vi "Display Module.vi"(7 "Callling VI":refnum<vi>) -> ()   [LabVIEW 2020]
uses:
  Display Module TypeDefs/IMAQ Z Scale Bar.ctl
  <vilib>/Utility/miscctls.llb/LVPointTypeDef.ctl
  <vilib>/vision/Image Controls.llb/IMAQ Image.ctl
  <vilib>/Utility/miscctls.llb/LVRectTypeDef.ctl
  Hardware Configuration/Hardware Configuration Controls/Standard Action.ctl
  <vilib>/event_ctls.llb/lveventtype.ctl
  Tools/TIFF Image Read and Write/ImageJ TIF Type Defs/TIF Write Image Information.ctl
  <vilib>/vision/NI_Vision_Development_Module.lvlib
panel:
  in  "Settings Menu":T1
  in  "Settings":bool
  in  "Refresh Rate (ms)":u32=30
  in  "Z Scale Channel 6":T2
  in  "Z Scale Channel 5":T2
  in  "Z Scale Channel 4":T2
  in  "Z Scale Channel 3":T2
  in  "Z Scale Channel 2":T2
  in  "Z Scale Channel 1":T2
  out "Messages":string
  in  "Max Left":bool
  in  "Max Right":bool
  in  "Add Display":bool
  in  "Remove Display":bool
  in  "Exit":bool
  out "Channel 6":T3(plugin-control)
  out "Channel 5":T3(plugin-control)
  out "Channel 4":T3(plugin-control)
  out "Channel 3":T3(plugin-control)
  out "Channel 2":T3(plugin-control)
  out "Channel 1":T3(plugin-control)
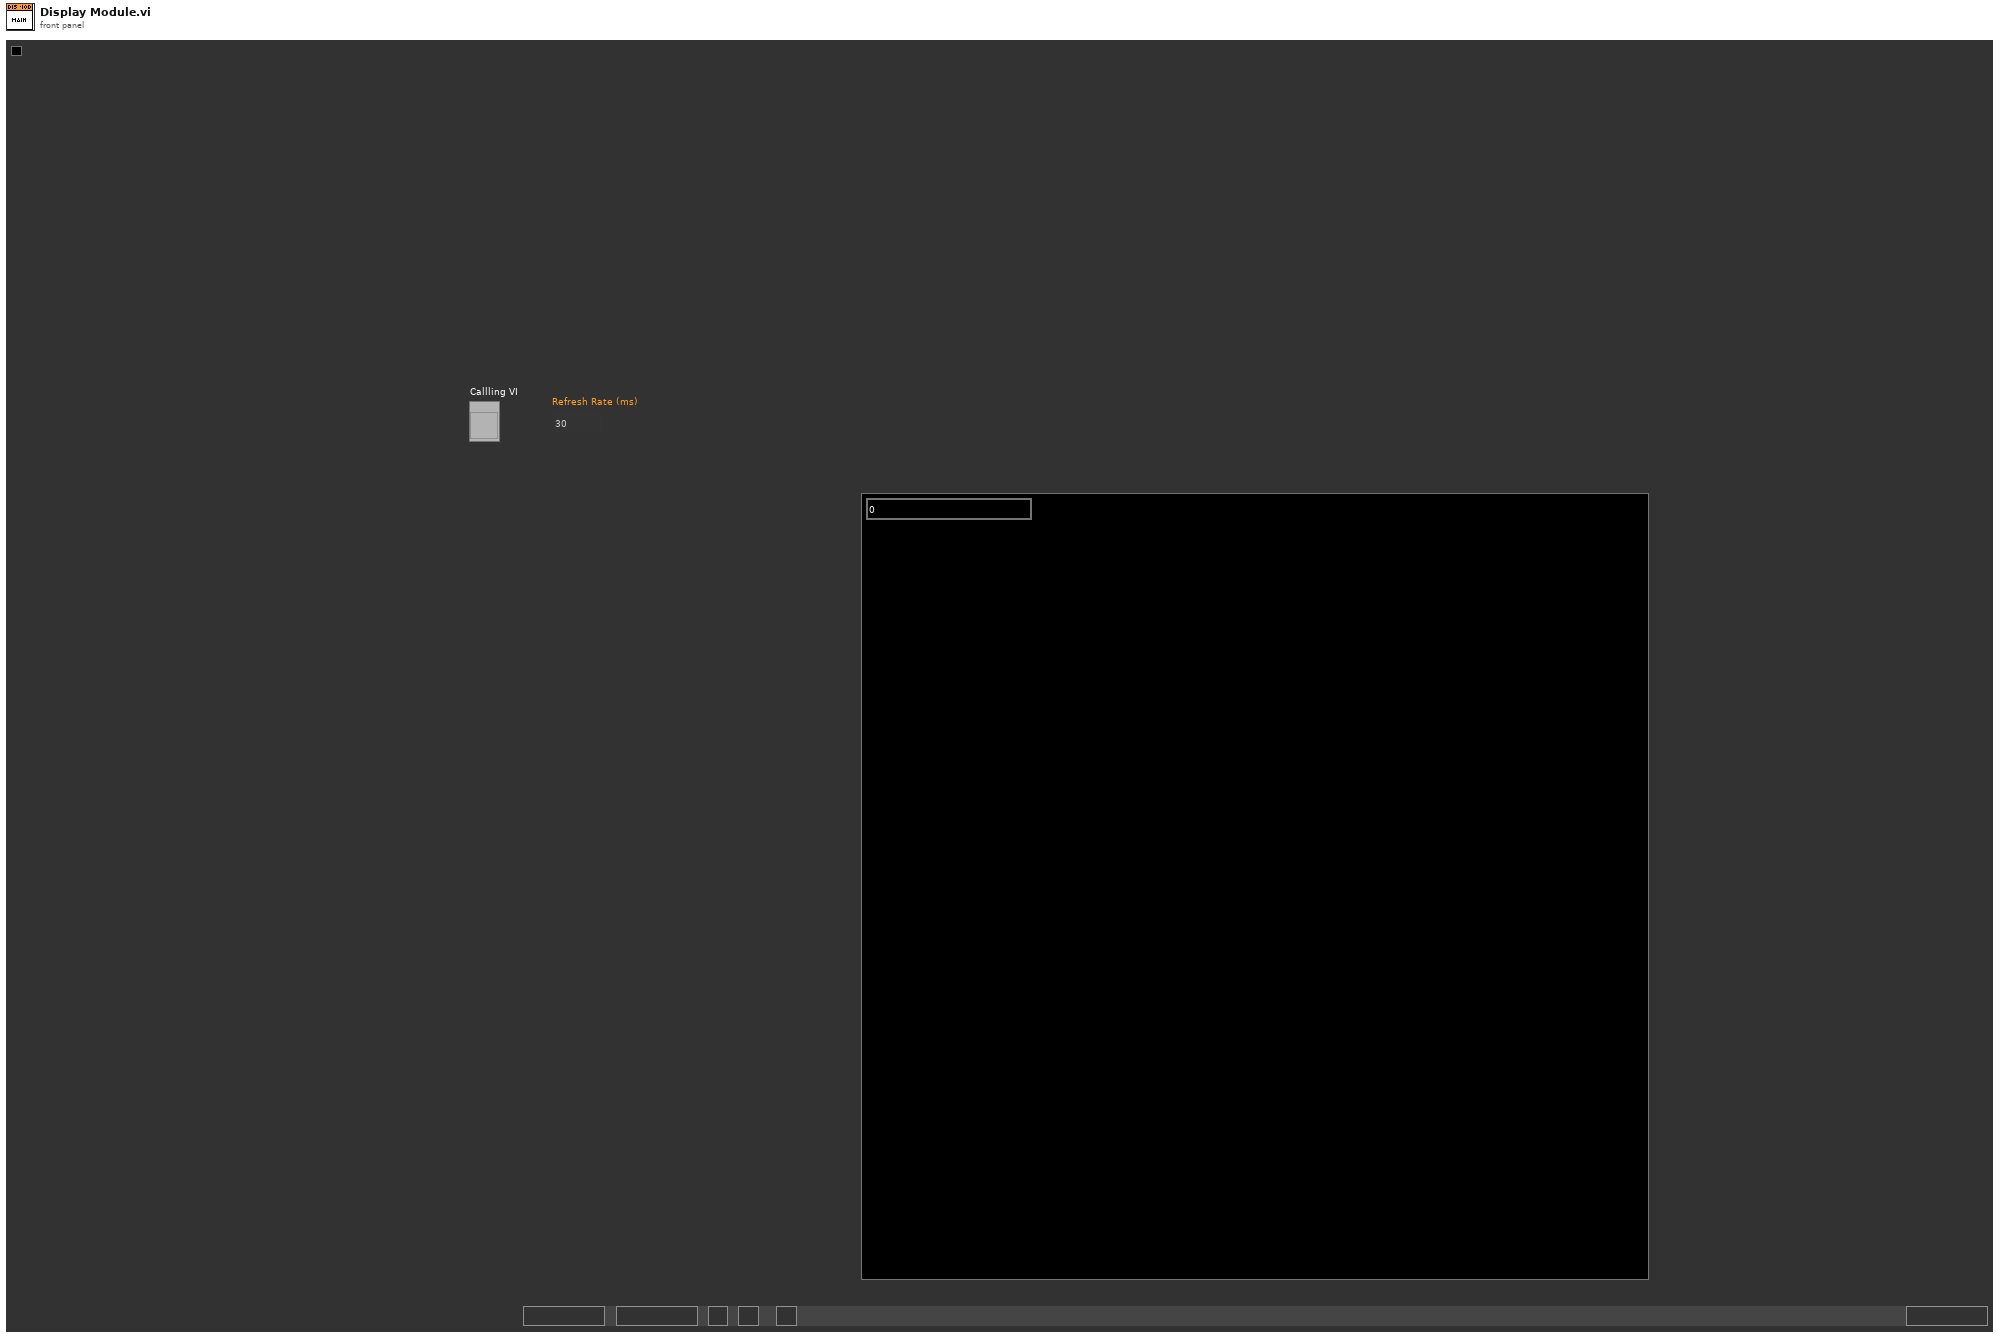
[diagram p1: front panel]
types:
  T1 = cluster{"Refresh Rate":bool, "Change Display Order":bool, "Display On / Off":bool}
  T2 = typedef "IMAQ Z Scale Bar.ctl" = cluster{"Z Scale Image":T3, "Z Scale Min":sgl, "Z Scale Max":sgl}
  T3 = typedef "IMAQ Image.ctl" = refnum<image>
  T4 = typedef "Image Type" = u32
  T5 = typedef "LVPointTypeDef.ctl" = cluster{"Horizontal":i16, "Vertical":i16}
  T6 = enum32{"Invalid", "Standard", "Closed", "Hidden", "Minimized", "Maximized"}
  T7 = enum16{"Always On", "Always Off", "Off While Running"}
  T8 = enum16{"Change Number", "Refresh Positions", "Get No. of Displays"}
  T9 = typedef "Standard Action.ctl" = enum16{"Read", "Write"}
  T10 = typedef "LVRectTypeDef.ctl" = cluster{"Left":i16, "Top":i16, "Right":i16, "Bottom":i16}
  T11 = typedef "lveventtype.ctl" = enum32{"Null", "Timeout", "Annotation Menu Selection", "Annotation Menu Selection?", "App Instance Close", "App Instance Close?", "Autoscale Range Change", "Bookmark Info Change", "Cell Edit", "Cell Edit?", "Cursor Grab", "Cursor Grab?", "Cursor Menu Selection", "Cursor Menu Selection?", "Cursor Move", "Cursor Release", "Data Change", "Direction Change", "Display State Change", "Drag Ended", "Drag Enter", "Drag Leave", "Drag Over", "Drag Source Update", "Drag Starting", "Drag Starting?", "Drop", "Exec State Change", "Key Down", "Key Down?", "Key Repeat", "Key Repeat?", "Key Up", "Listbox Double Click", "Menu Activation?", "Menu Selection (App)", "Menu Selection? (App)", "Menu Selection (User)", "Mouse Down", "Mouse Down?", "Mouse Enter", "Mouse Leave", "Mouse Move", "Mouse Up", "Mouse Wheel", "NI Security User Change (App)", "Pane Size", "Panel Close", "Panel Close?", "Panel Resize", "Plot Attribute Change", "Scale Range Change", "Shortcut Menu Activation?", "Shortcut Menu Selection (App)", "Shortcut Menu Selection? (App)", "Shortcut Menu Selection (User)", "Tree Double Click", "Tree Drag", "Tree Drag?", "Tree Drop", "Tree Drop?", "Tree Item Close", "Tree Item Close?", "Tree Item Open", "Tree Item Open?", "User Event", "Value Change"}
  T12 = cluster{"Global Rectangle":i32[], "Contours":cluster{"Contour Type":u32, "ROI Type":u32, "Points":i32[]}[]}
  T13 = typedef "TIF Write Image Information.ctl" = cluster{"Image Width (Pixels)":u32, "Image Height (Pixels)":u32, "Pixel Width (µm)":dbl, "Pixel Height (µm)":dbl, "Bits Per Sample (e.g. 16)":u32, "No. of Frames":u32, "No. of Slices":u32, "Time Step (sec)":dbl, "Z Step (µm)":dbl}
  T14 = typedef "LVAllMonitorsDisplayTypeDef.ctl" = cluster{"Bounds":cluster{"Left":i16, "Top":i16, "Right":i16, "Bottom":i16}, "Depth":i16}[]
  T15 = cluster{"Bounds":cluster{"Left":i16, "Top":i16, "Right":i16, "Bottom":i16}, "Depth":i16}
  T16 = cluster{"Mean Value":sgl, "Standard Variation":sgl, "Minimal Value":sgl, "Maximal Value":sgl, "Area (calibrated)":sgl, "Area (pixels)":u32, "%":sgl, "Calibration Valid":bool}
  T17 = enum16{"big-endian, network order", "native, host order", "little-endian"}
  T18 = cluster{"Contour Type":u32, "ROI Type":u32, "Points":i32[]}[]
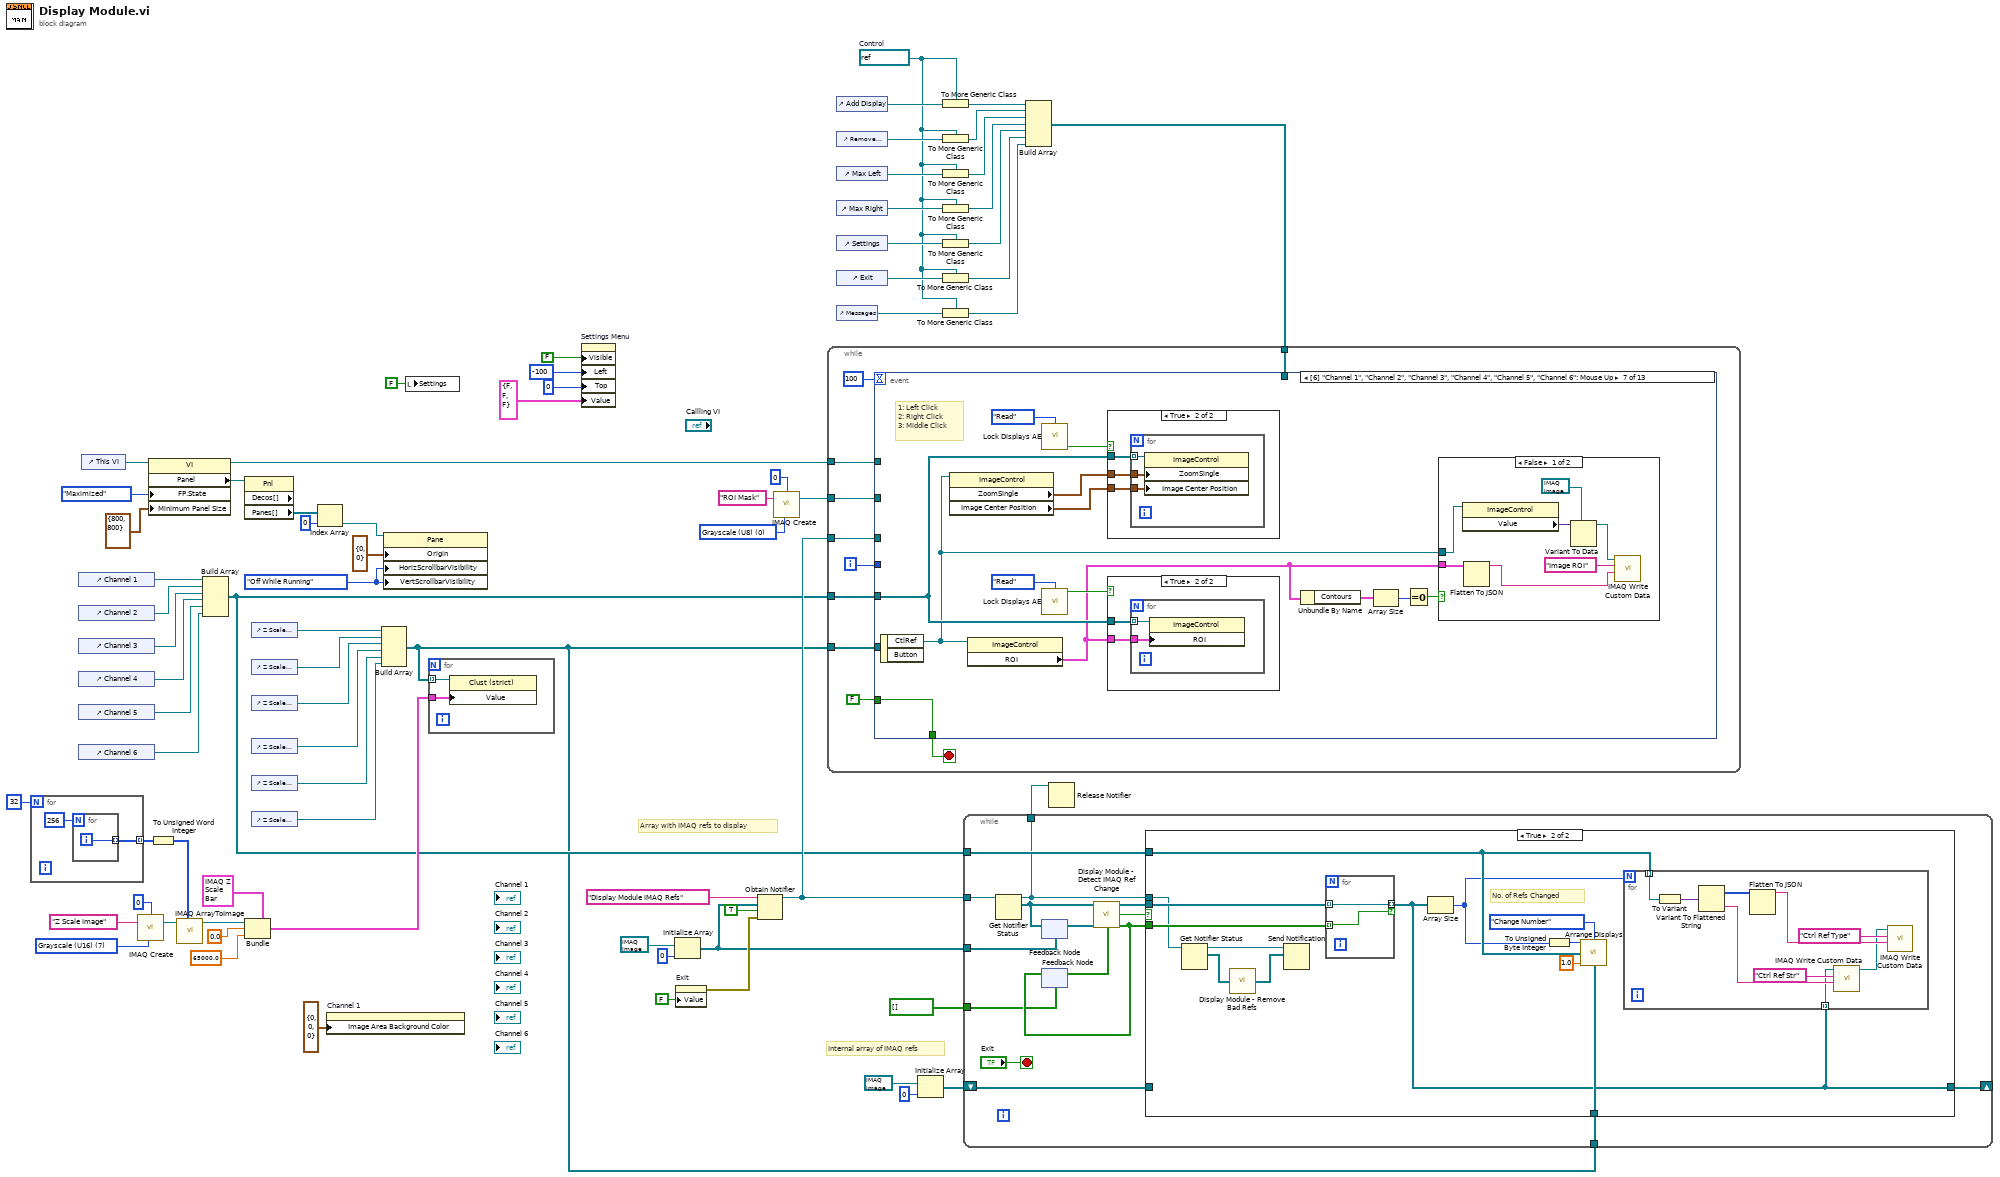
[diagram p0: block diagram]
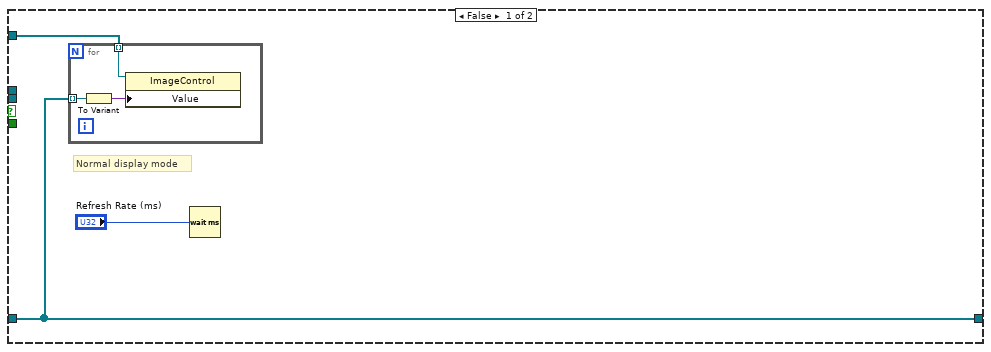
[diagram p2: hidden frame]
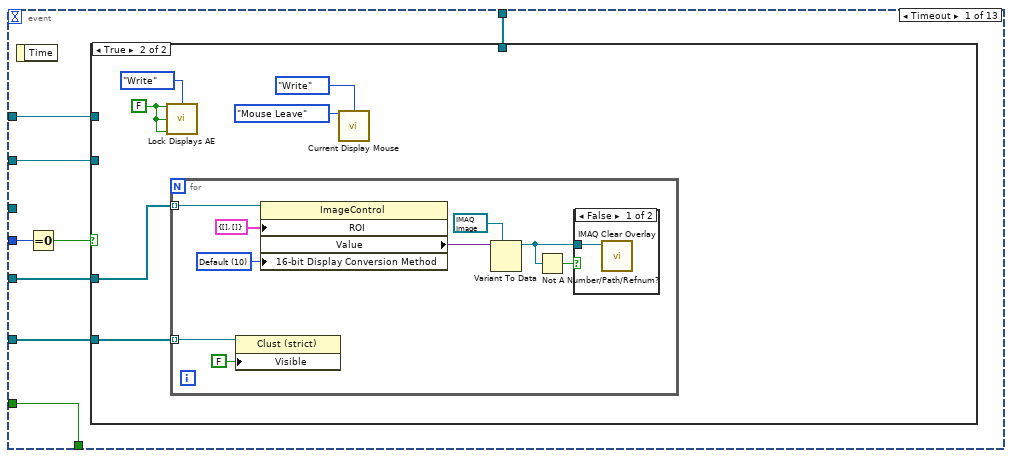
[diagram p3: hidden frame]
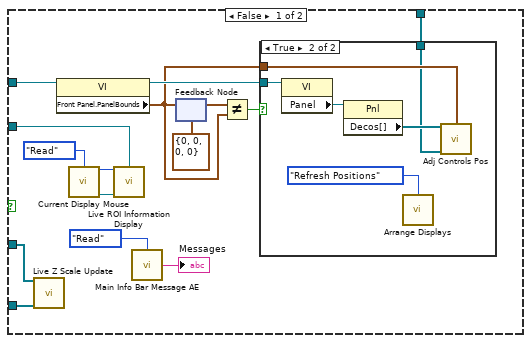
[diagram p4: hidden frame]
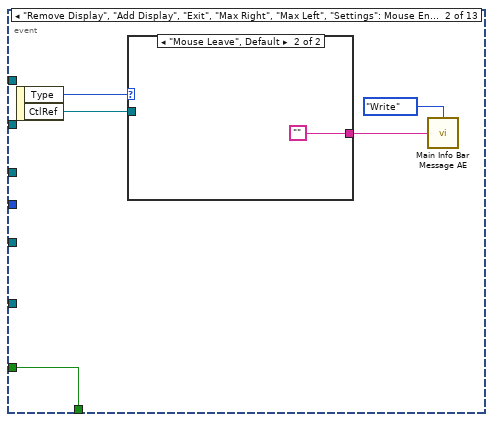
[diagram p7: hidden frame]
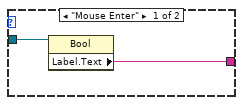
[diagram p8: hidden frame]
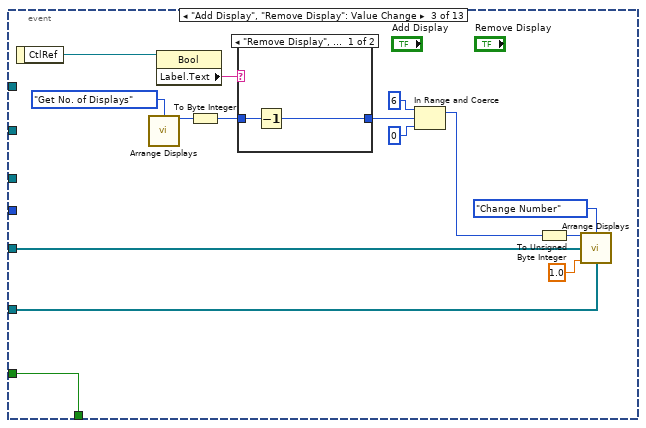
[diagram p9: hidden frame]
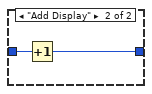
[diagram p10: hidden frame]
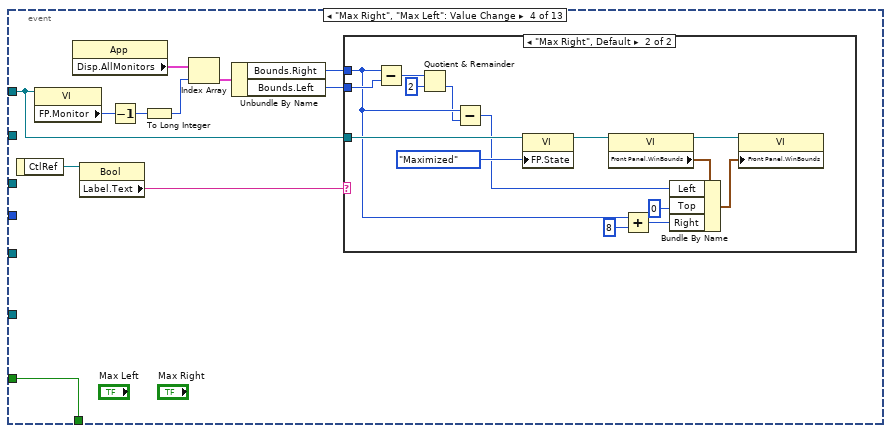
[diagram p11: hidden frame]
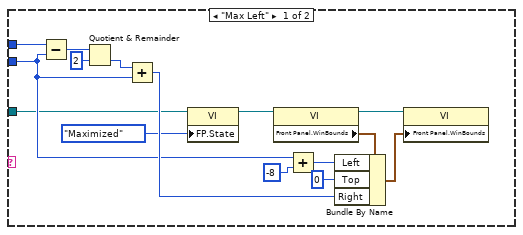
[diagram p12: hidden frame]
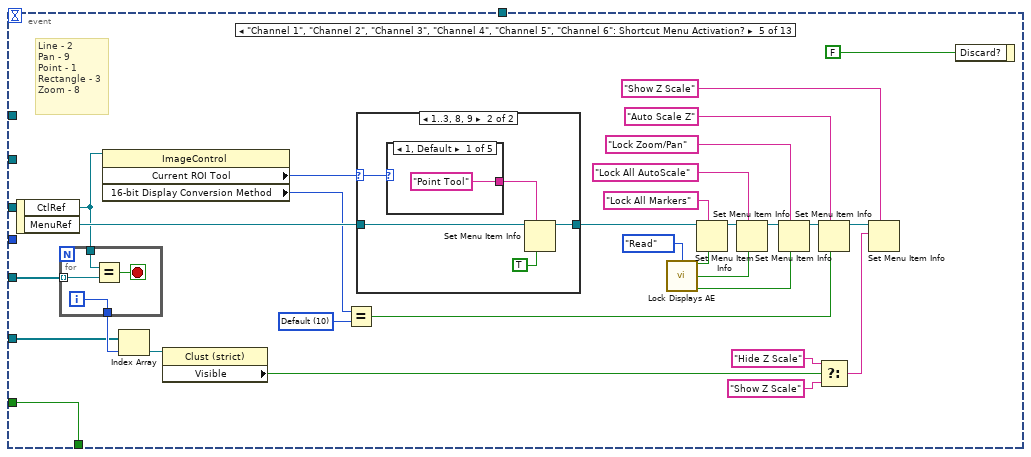
[diagram p13: hidden frame]
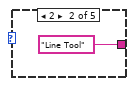
[diagram p15: hidden frame]
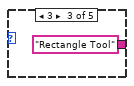
[diagram p16: hidden frame]
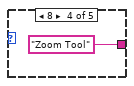
[diagram p17: hidden frame]
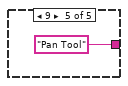
[diagram p18: hidden frame]
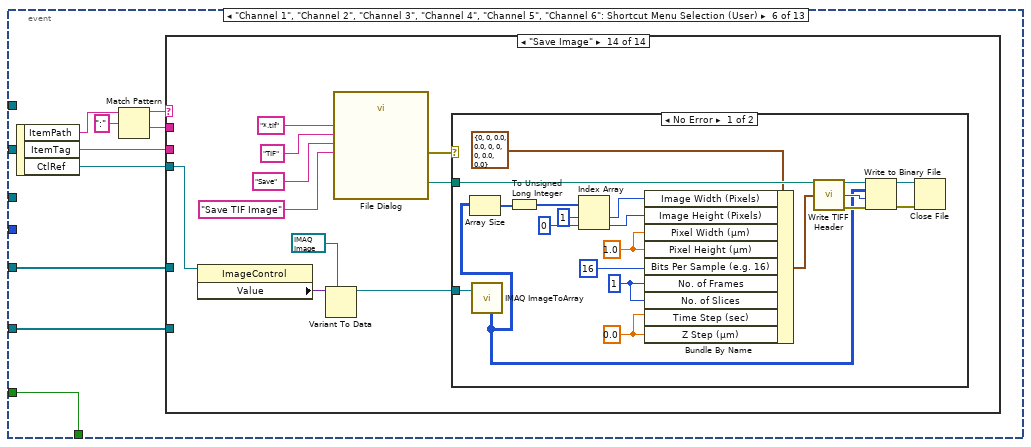
[diagram p19: hidden frame]
diagram:
  w23 = refnum<vi> refnum  # Control
  w47 = T4 7 items=["Grayscale (U8)", "Grayscale (I16)", "Grayscale (SGL)", "Complex (CSG)", "RGB (U32)", "HSL (U32)", "RGB (U64)", "Grayscale (U16)"] ("Image Type")
  w53 = T4 0 items=["Grayscale (U8)", "Grayscale (I16)", "Grayscale (SGL)", "Complex (CSG)", "RGB (U32)", "HSL (U32)", "RGB (U64)", "Grayscale (U16)"] ("Image Type")
  w66 = T7."Off While Running" ("Vertical Scrollbar Visibility")
  # "Internal array of IMAQ refs"
  # "Array with IMAQ refs to display"
  n1 = for {
    N: 32 -> [_]
    tunnel: [w76] -> w45 mode=indexing
    n2 = for {
      N: 256 -> [_]
      tunnel: [w78] -> w76 mode=indexing
      i -> [w78]
    }
  }
  n3 = control-ref of="Channel 1"() -> (w75:refnum<vi>)
  n4 = control-ref of="Channel 2"() -> (w70:refnum<vi>)
  n5 = control-ref of="Channel 3"() -> (w71:refnum<vi>)
  n6 = control-ref of="Channel 4"() -> (w72:refnum<vi>)
  n7 = control-ref of="Channel 5"() -> (w73:refnum<vi>)
  n8 = control-ref of="Channel 6"() -> (w74:refnum<vi>)
  n9 = control-ref of="This VI"() -> (w65:refnum<vi>)
  n10 = call "IMAQ Create"("Border Size"=0, "Image Name"="Z Scale Image", "Image Type"=w47) -> ("New Image"=w46:T3)  [unwired: 2 in, 1 out]
  n11 = property class="VI"(reference=w65, "FP.State"=T6."Maximized" ("Front Panel Window:State"), "Minimum Panel Size"=T5 {"Horizontal"=800, "Vertical"=800} ("Front Panel Window:Minimum Size")) -> (reference out=w60:refnum<vi>, "Panel"=w61:refnum<vi>)  [unwired: 1 in, 1 out]
  n12 = To Unsigned Word Integer(number=w45) -> (unsigned 16bit integer=w44:u16[][])
  n13 = call "IMAQ ArrayToImage"("Image Pixels (U16)"=w44, "Image"=w46) -> ("Image Out"=w43:T3)  [unwired: 8 in, 1 out]
  n14 = Build Array(w75, w70, w71, w72, w73, w74) -> (w3:refnum<vi>[])
  n15 = property class="Pnl" props=["Decos[]", "Panes[]"](reference=w61) -> ("Panes[]"=w62:refnum<vi>[])  [unwired: 1 in, 3 out]
  n16 = Bundle(cluster=T2 {"Z Scale Image"="remote image 000001BB3853FFD8", "Z Scale Min"=0.0, "Z Scale Max"=65000.0} ("Z Scale Channel 6"), "Z Scale Image"=w43, "Z Scale Min"=sgl 0.0, "Z Scale Max"=sgl 65000.0) -> (w35:T2)
  n17 = control-ref of="Z Scale Channel 1"() -> (w1:refnum<vi>)
  n18 = control-ref of="Z Scale Channel 2"() -> (w36:refnum<vi>)
  n19 = control-ref of="Z Scale Channel 3"() -> (w37:refnum<vi>)
  n20 = control-ref of="Z Scale Channel 4"() -> (w38:refnum<vi>)
  n21 = control-ref of="Z Scale Channel 5"() -> (w39:refnum<vi>)
  n22 = control-ref of="Z Scale Channel 6"() -> (w40:refnum<vi>)
  n23 = Index Array(array=w62, index=0) -> (element=w68:refnum<vi>)
  n24 = property on="Channel 1" class="ImageControl"("Image Area Background Color"=cluster{"Red":u8, "Green":u8, "Blue":u8} {"Red"=0, "Green"=0, "Blue"=0} ("Image Area:Background:Background Color")) -> ()  [unwired: 2 in, 2 out]
  n25 = Build Array(w1, w36, w37, w38, w39, w40) -> (w2:refnum<vi>[])
  n26 = property class="Pane"(reference=w68, "Origin"=T5 {"Horizontal"=0, "Vertical"=0}, "HorizScrollbarVisibility"=w66, "VertScrollbarVisibility"=w66) -> ()  [unwired: 1 in, 2 out]
  n27 = local write "Settings"(FALSE ("Settings")) -> ()
  n28 = for {
    tunnel: w2 -> [w80] mode=indexing
    tunnel: w35 -> [w79]
    n29 = property class="Clust (strict)"(reference=w80, "Value"=w79) -> ()  [unwired: 1 in, 2 out]
  }
  n30 = property on="Settings Menu" class="Clust (strict)"("Visible"=FALSE, "Left"=-100 ("Position:Left"), "Top"=0 ("Position:Top"), "Value"=T1 {"Refresh Rate"=FALSE, "Change Display Order"=FALSE, "Display On / Off"=FALSE} ("Settings Menu")) -> ()  [unwired: 2 in, 2 out]
  n31 = Initialize Array(T3 refnum ("New Image"), 0 ("dimension size")) -> (w6:T3[])
  n32 = property on="Exit" class="Bool (strict)"("Value"=FALSE ("Exit")) -> (error out=w31:errorcluster)  [unwired: 2 in, 1 out]
  n33 = Obtain Notifier(name (unnamed)="Display Module IMAQ Refs", notification data type=w6, create if not found? (T)=TRUE, error in (no error)=w31) -> (notifier out=w5:refnum<notifier>)  [unwired: 2 out]
  n34 = call "IMAQ Create"("Border Size"=0, "Image Name"="ROI Mask", "Image Type"=w53) -> ("New Image"=w51:T3)  [unwired: 2 in, 1 out]
  n35 = control-ref of="Add Display"() -> (w30:refnum<vi>)
  n36 = control-ref of="Remove Display"() -> (w24:refnum<vi>)
  n37 = control-ref of="Max Left"() -> (w25:refnum<vi>)
  n38 = control-ref of="Max Right"() -> (w26:refnum<vi>)
  n39 = control-ref of="Settings"() -> (w27:refnum<vi>)
  n40 = control-ref of="Exit"() -> (w28:refnum<vi>)
  n41 = control-ref of="Messages"() -> (w29:refnum<vi>)
  n42 = Initialize Array(T3 refnum ("New Image"), 0 ("dimension size")) -> (w7:T3[])
  n43 = To More Generic Class(target class=w23, reference=w30) -> (generic class reference=w22:refnum<vi>)
  n44 = To More Generic Class(target class=w23, reference=w24) -> (generic class reference=w21:refnum<vi>)
  n45 = To More Generic Class(target class=w23, reference=w25) -> (generic class reference=w20:refnum<vi>)
  n46 = To More Generic Class(target class=w23, reference=w26) -> (generic class reference=w19:refnum<vi>)
  n47 = To More Generic Class(target class=w23, reference=w27) -> (generic class reference=w18:refnum<vi>)
  n48 = To More Generic Class(target class=w23, reference=w28) -> (generic class reference=w17:refnum<vi>)
  n49 = To More Generic Class(target class=w23, reference=w29) -> (generic class reference=w16:refnum<vi>)
  n50 = while {
    tunnel: w5 -> [w95]
    tunnel: w3 -> [w94]
    tunnel: [w84] -> w55
    tunnel: w2 -> [w92]
    shift-right: [w85] -> _
    shift-left: w7 -> [w91]
    tunnel: w6 -> [w88]
    tunnel: bool[] [] -> [w81]
    stop <- "Exit" stop-if-true
    n51 = Get Notifier Status(notifier=w95) -> (notifier out=w84:refnum<notifier>, current notification=w90:T3[])  [unwired: 1 in, 3 out]
    n52 = feedback-in #1(w90) -> ()
    n53 = feedback #1(w88) -> (w89:T3[])
    n54 = feedback #2(w81) -> (w82:bool[])
    n55 = call "Display Module - Detect IMAQ Ref Change.vi"("Current Image Refs"=w90, "Previous Image Refs"=w89, "Previous Image Display Flags"=w82) -> ("Current Image Refs (Dup)"=w87:T3[], "Change Detected"=w86:bool, "Image Display Flags"=w83:bool[])  [unwired: 10 in]
    n56 = feedback-in #2(w83) -> ()
    n57 = case shown="True" w86 {
      tunnel: w87 -> [_ w110]
      tunnel: w94 -> [w98 w104]
      tunnel: w92 -> [_ w112]
      tunnel: w91 -> [w96 _]
      tunnel: w83 -> [_ w109]
      tunnel: [w96 w102] -> w85
      tunnel: w84 -> [_ w105]
      frame False {
        # "Normal display mode"
        n58 = for {
          tunnel: w98 -> [w101] mode=indexing
          tunnel: w96 -> [w99] mode=indexing
          n59 = To Variant(anything=w99) -> (Variant=w100:variant)
          n60 = property class="ImageControl"(reference=w101, "Value"=w100) -> ()  [unwired: 1 in, 2 out]
        }
        n61 = Wait (ms)(milliseconds to wait="Refresh Rate (ms)") -> ()  [unwired: 1 out]
      }
      frame True {
        # "No. of Refs Changed"
        n62 = Get Notifier Status(notifier=w105) -> (notifier out=w107:refnum<notifier>, current notification=w106:T3[])  [unwired: 1 in, 3 out]
        n63 = call "Display Module - Remove Bad Refs.vi"("Image Refs In"=w106) -> ("Image Refs Out"=w108:T3[])  [unwired: 14 in]
        n64 = Send Notification(notification=w108, notifier=w107) -> ()  [unwired: 1 in, 2 out]
        n65 = for {
          tunnel: w110 -> [w125] mode=indexing
          tunnel: [w125] -> w102 mode=indexing if=w124
          tunnel: w109 -> [w124] mode=indexing
        }
        n66 = Array Size(array=w102) -> (size(s)=w103:i32)
        n67 = To Unsigned Byte Integer(number=w103) -> (unsigned 8bit integer=w114:u8)
        n68 = call "Arrange Displays.vi"("Number of Displays"=w114, "Action"=T8."Change Number", "IMAQ Display Refs"=w104, "Aspect Ratio (Width/Height)"=1.0, "Z Scale Refs"=w112) -> ()  [unwired: 9 in, 2 out]
        n69 = for {
          N: w103 -> [_]
          tunnel: w104 -> [w122] mode=indexing
          tunnel: w102 -> [w115] mode=indexing
          n70 = To Variant(anything=w122) -> (Variant=w123:variant)
          n71 = Variant To Flattened String(Variant=w123) -> (data string=w117:string, 1:w120:i16[])
          n72 = Flatten To JSON(anything=w120) -> (JSON string=w118:string)  [unwired: 2 in, 1 out]
          n73 = call "IMAQ Write Custom Data"("Custom Data In"=w117, "Key"="Ctrl Ref Str", "Image"=w115) -> ("Image Out"=w116:T3)  [unwired: 7 in, 1 out]
          n74 = call "IMAQ Write Custom Data"("Custom Data In"=w118, "Key"="Ctrl Ref Type", "Image"=w116) -> ()  [unwired: 7 in, 2 out]
        }
      }
    }
  }
  n75 = Build Array(w22, w21, w20, w19, w18, w17, w16) -> (w15:refnum<vi>[])
  n76 = while {
    tunnel: w3 -> [w134]
    tunnel: w60 -> [w130]
    tunnel: w51 -> [w129]
    tunnel: w2 -> [w128]
    tunnel: w15 -> [w127]
    tunnel: w5 -> [w126]
    i -> [w135]
    stop <- w133 stop-if-true
    n77 = event shown="[6] \"Channel 1\", \"Channel 2\", \"Channel 3\", \"Channel 4\", \"Channel 5\", \"Channel 6\": Mouse Up" {
      selector: _ -> [_ _ _ _ _ _ _ _ _ _ _ _ _]
      dyn-events: _ -> [_ _ _ _ _ _ _ _ _ _ _ _ _]
      timeout: 100 -> [_ _ _ _ _ _ _ _ _ _ _ _ _]
      tunnel: w135 -> [w143 _ _ _ _ _ _ _ _ _ _ _ _]
      tunnel: w134 -> [w141 _ w190 _ w253 w296 w496 _ w532 w540 _ w567 w603]
      tunnel: [w140 w185 w203 w218 w277 w302 w501 w523 w534 w546 w556 w579 w604] -> w133
      tunnel: FALSE -> [w140 w185 w203 w218 w277 w302 w501 w523 w534 w546 w556 w579 _]
      tunnel: w130 -> [w139 _ _ w209 _ _ _ _ _ _ _ _ _]
      tunnel: w129 -> [w138 _ _ _ _ _ _ _ _ _ _ _ w602]
      tunnel: w128 -> [w137 _ w191 _ w254 w295 _ _ w533 _ _ _ _]
      tunnel: w127 -> [w136 _ _ _ _ _ _ _ _ _ _ _ _]
      tunnel: w126 -> [_ _ _ _ _ _ _ _ _ _ _ w568 _]
      event Timeout {
        n78 = event-data() -> ()  [unwired: 1 in, 1 out]
        n79 = Equal To 0?(x=w143) -> (x = 0?=w142:bool)
        n80 = case shown="True" w142 {
          tunnel: w141 -> [w146 w168]
          tunnel: w139 -> [w158 _]
          tunnel: w138 -> [w152 _]
          tunnel: w137 -> [w145 w167]
          tunnel: w136 -> [w144 _]
          frame False {
            n81 = call "Live Z Scale Update.vi"("IMAQ Display Refs"=w146, "Z Scale Refs"=w145) -> ()  [unwired: 14 in]
            n82 = property class="VI"(reference=w158) -> (reference out=w154:refnum<vi>, "Front Panel.PanelBounds"=w153:T10)  [unwired: 1 in, 1 out]
            n83 = call "Current Display Mouse.vi"("Action"=Standard_Action."Read") -> ("Event Type Out"=w150:T11, "IMAQ Image Display Ref Out"=w149:refnum<vi>)  [unwired: 13 in]
            n84 = call "Live ROI Information Display.vi"("Event Type"=w150, "ROI Mask REF"=w152, "IMAQ Image Display Ref"=w149) -> ()  [unwired: 13 in]
            n85 = call "Main Info Bar Message AE.vi"("Action"=Standard_Action."Read") -> ("Message Out"=→"Messages":string)  [unwired: 14 in]
            n86 = feedback-in #3(w153) -> ()
            n87 = feedback #3(T10 {"Left"=0, "Top"=0, "Right"=0, "Bottom"=0} ("Front Panel.PanelBounds")) -> (w157:T10)
            n88 = Not Equal?(x=w157, y=w153) -> (x != y?=w155:bool)
            n89 = case shown="True" w155 {
              tunnel: w154 -> [_ w162]
              tunnel: w153 -> [_ w161]
              tunnel: w144 -> [_ w160]
              frame False {
              }
              frame True {
                n90 = property class="VI"(reference=w162) -> ("Panel"=w164:refnum<vi>)  [unwired: 1 in, 2 out]
                n91 = property class="Pnl"(reference=w164) -> ("Decos[]"=w163:refnum<vi>[])  [unwired: 1 in, 2 out]
                n92 = call "Arrange Displays.vi"("Action"=T8."Refresh Positions") -> ()  [unwired: 13 in, 2 out]
                n93 = call "Adj Controls Pos.vi"("Decoration Ref Array"=w163, "Panel Bounds"=w161, "Control Ref Array"=w160) -> ()  [unwired: 13 in]
              }
            }
          }
          frame True {
            w170 = FALSE ("Lock All Markers")
            n94 = call "Lock Displays AE.vi"("Lock All Markers"=w170, "Action"=Standard_Action."Write", "Lock All AutoScale"=w170, "Lock Pan/Zoom"=w170) -> ()  [unwired: 9 in, 3 out]
            n95 = for {
              tunnel: w168 -> [w174] mode=indexing
              tunnel: w167 -> [w173] mode=indexing
              w171 = u32 10 items=["Default"=10, "Most Significant Bits"=11, "Full Dynamic"=12, "Downshift"=13, "Given Range"=14, "90% Dynamic"=15, "Given Percent Range"=16] ("16-bit Display Mapping:Conversion Method")
              n96 = property class="Clust (strict)"(reference=w173, "Visible"=FALSE) -> ()  [unwired: 1 in, 2 out]
              n97 = property class="ImageControl"(reference=w174, "ROI"=T12 {"Global Rectangle"=[], "Contours"=[]}, "16-bit Display Conversion Method"=w171) -> ("Value"=w175:variant)  [unwired: 1 in, 2 out]
              n98 = Variant To Data(type=T3 refnum ("New Image"), Variant=w175) -> (data=w178:T3)  [unwired: 1 in, 1 out]
              n99 = Not A Number/Path/Refnum?(number/path/refnum=w178) -> (NaN/Path/Refnum?=w177:bool)
              n100 = case shown="False" w177 {
                tunnel: w178 -> [w180 _]
                frame False {
                  n101 = call "IMAQ Clear Overlay"("Image"=w180) -> ()  [unwired: 9 in, 2 out]
                }
                frame True {
                }
              }
            }
            n102 = call "Current Display Mouse.vi"("Event Type"=lveventtype."Mouse Leave", "Action"=Standard_Action."Write") -> ()  [unwired: 12 in, 2 out]
          }
        }
      }
      event "Remove Display", "Add Display", "Exit", "Max Right", "Max Left", "Settings", "Settings Menu.Refresh Rate", "Settings Menu.Change Display Order", "Settings Menu.Display On / Off": Mouse Enter; "Remove Display", "Add Display", "Exit", "Max Right", "Max Left", "Settings", "Settings Menu.Refresh Rate", "Settings Menu.Change Display Order", "Settings Menu.Display On / Off": Mouse Leave {
        n103 = event-data() -> ("Type"=w184:T11, "CtlRef"=w183:refnum<vi>)  [unwired: 1 in]
        n104 = case shown="\"Mouse Leave\", Default" w184 {
          tunnel: w183 -> [w187 _]
          tunnel: [w186 ""] -> w181
          frame "Mouse Enter" {
            n105 = property class="Bool"(reference=w187) -> ("Label.Text"=w186:string)  [unwired: 1 in, 2 out]
          }
          frame "Mouse Leave", Default {
          }
        }
        n106 = call "Main Info Bar Message AE.vi"("Action"=Standard_Action."Write", "Message"=w181) -> ()  [unwired: 13 in, 1 out]
      }
      event "Add Display", "Remove Display": Value Change {
        n107 = event-data() -> ("CtlRef"=w202:refnum<vi>)  [unwired: 1 in]
        n108 = call "Arrange Displays.vi"("Action"=T8."Get No. of Displays") -> ("Number of Displays Out"=w193:u8)  [unwired: 13 in, 1 out]
        n109 = property class="Bool"(reference=w202) -> ("Label.Text"=w201:string)  [unwired: 1 in, 2 out]
        n110 = To Byte Integer(number=w193) -> (8bit integer=w192:i8)
        n111 = case shown="\"Remove Display\", Default" w201 {
          tunnel: w192 -> [w205 w207]
          tunnel: [w204 w206] -> w198
          frame "Remove Display", Default {
            n112 = Decrement(x=w205) -> (x-1=w204:i8)
          }
          frame "Add Display" {
            n113 = Increment(x=w207) -> (x+1=w206:i8)
          }
        }
        n114 = In Range and Coerce(upper limit=i8 6, x=w198, lower limit=i8 0) -> (coerced(x)=w197:i8)  [unwired: 1 out]
        n115 = To Unsigned Byte Integer(number=w197) -> (unsigned 8bit integer=w196:u8)
        n116 = call "Arrange Displays.vi"("Number of Displays"=w196, "Action"=T8."Change Number", "IMAQ Display Refs"=w190, "Aspect Ratio (Width/Height)"=1.0, "Z Scale Refs"=w191) -> ()  [unwired: 9 in, 2 out]
      }
      event "Max Right", "Max Left": Value Change {
        n117 = event-data() -> ("CtlRef"=w217:refnum<vi>)  [unwired: 1 in]
        n118 = property class="VI"(reference=w209) -> ("FP.Monitor"=w216:u16)  [unwired: 1 in, 2 out]
        n119 = property class="App"() -> ("Disp.AllMonitors"=w215:T14)  [unwired: 2 in, 2 out]
        n120 = property class="Bool"(reference=w217) -> ("Label.Text"=w208:string)  [unwired: 1 in, 2 out]
        n121 = Decrement(x=w216) -> (x-1=w214:u16)
        n122 = To Long Integer(number=w214) -> (32bit integer=w213:i32)
        n123 = Index Array(array=w215, index=w213) -> (element=w212:T15)
        n124 = Unbundle By Name(w212) -> ("Bounds.Right"=w211:i16, "Bounds.Left"=w210:i16)
        n125 = case shown="\"Max Right\", Default" w208 {
          tunnel: w211 -> [w233 w236]
          tunnel: w210 -> [w221 w240]
          tunnel: w209 -> [w219 w239]
          frame "Max Left" {
            n126 = Subtract(x=w233, y=w221) -> (x-y=w228:i16)
            n127 = Quotient & Remainder(x=w228, y=i16 2) -> (floor(x/y)=w226:i16)  [unwired: 1 out]
            n128 = Add(x=w226, y=w221) -> (x+y=w225:i16)
            n129 = property class="VI"(reference=w219, "FP.State"=T6."Maximized" ("Front Panel Window:State")) -> (reference out=w223:refnum<vi>)  [unwired: 1 in, 1 out]
            n130 = property class="VI"(reference=w223) -> (reference out=w232:refnum<vi>, "Front Panel.WinBounds"=w230:T10)  [unwired: 1 in, 1 out]
            n131 = Add(x=w221, y=i16 -8 ("Left")) -> (x+y=w220:i16)
            n132 = Bundle By Name(cluster=w230, "Left"=w220, "Top"=i16 0, "Right"=w225) -> (w231:T10)
            n133 = property class="VI"(reference=w232, "Front Panel.WinBounds"=w231) -> ()  [unwired: 1 in, 2 out]
          }
          frame "Max Right", Default {
            n134 = Subtract(x=w236, y=w240) -> (x-y=w245:i16)
            n135 = Quotient & Remainder(x=w245, y=i16 2) -> (floor(x/y)=w235:i16)  [unwired: 1 out]
            n136 = Subtract(x=w236, y=w235) -> (x-y=w234:i16)
            n137 = property class="VI"(reference=w239, "FP.State"=T6."Maximized" ("Front Panel Window:State")) -> (reference out=w242:refnum<vi>)  [unwired: 1 in, 1 out]
            n138 = property class="VI"(reference=w242) -> (reference out=w248:refnum<vi>, "Front Panel.WinBounds"=w246:T10)  [unwired: 1 in, 1 out]
            n139 = Add(x=w236, y=i16 8 ("Left")) -> (x+y=w237:i16)
            n140 = Bundle By Name(cluster=w246, "Left"=w234, "Top"=i16 0, "Right"=w237) -> (w247:T10)
            n141 = property class="VI"(reference=w248, "Front Panel.WinBounds"=w247) -> ()  [unwired: 1 in, 2 out]
          }
        }
      }
      event "Channel 1", "Channel 2", "Channel 3", "Channel 4", "Channel 5", "Channel 6": Shortcut Menu Activation? {
        w260 = u32 10 items=["Default"=10, "Most Significant Bits"=11, "Full Dynamic"=12, "Downshift"=13, "Given Range"=14, "90% Dynamic"=15, "Given Percent Range"=16] ("16-bit Display Mapping:Conversion Method")
        # "Line - 2\nPan - 9\nPoint - 1\nRectangle - 3\nZoom - 8"
        n142 = event-data() -> ("CtlRef"=w255:refnum<vi>, "MenuRef"=w275:refnum<k9>)  [unwired: 1 in]
        n143 = for {
          tunnel: w253 -> [w282] mode=indexing
          tunnel: w255 -> [w280]
          tunnel: [w279] -> w257
          i -> [w279]
          stop <- w281 stop-if-true
          n144 = Equal?(x=w280, y=w282) -> (x = y?=w281:bool)
        }
        n145 = property class="ImageControl"(reference=w255) -> ("Current ROI Tool"=w276:u32, "16-bit Display Conversion Method"=w262:u32)  [unwired: 1 in, 2 out]
        n146 = Index Array(array=w254, index=w257) -> (element=w256:refnum<vi>)
        n147 = property class="Clust (strict)"(reference=w256) -> ("Visible"=w249:bool)  [unwired: 1 in, 2 out]
        n148 = Equal?(x=w262, y=w260) -> (x = y?=w261:bool)
        n149 = case shown="1..3, 8, 9" w276 {
          selector: w276 -> [_ w288]
          tunnel: w275 -> [w283 w286]
          tunnel: [w283 w284] -> w274
          frame Default {
          }
          frame 1..3, 8, 9 {
            n150 = case shown="1, Default" w288 {
              tunnel: ["Point Tool" ("item tag") "Line Tool" ("item tag") "Rectangle Tool" ("item tag") "Zoom Tool" ("item tag") "Pan Tool" ("item tag")] -> w285
              frame 1, Default {
              }
              frame 2 {
              }
              frame 3 {
              }
              frame 8 {
              }
              frame 9 {
              }
            }
            n151 = Set Menu Item Info(6:TRUE ("checked"), 7:w285, 11:w286) -> (3:w284:refnum<k9>)  [unwired: 4 in, 1 out]
          }
        }
        n152 = call "Lock Displays AE.vi"("Action"=Standard_Action."Read") -> ("Lock All Markers Out"=w267:bool, "Lock All AutoScale Out"=w266:bool, "Lock Pan/Zoom Out"=w265:bool)  [unwired: 12 in]
        n153 = Set Menu Item Info(6:w267, 7:"Lock All Markers" ("item tag"), 11:w274) -> (3:w273:refnum<k9>)  [unwired: 4 in, 1 out]
        n154 = Set Menu Item Info(6:w266, 7:"Lock All AutoScale" ("item tag"), 11:w273) -> (3:w272:refnum<k9>)  [unwired: 4 in, 1 out]
        n155 = Set Menu Item Info(6:w265, 7:"Lock Zoom/Pan" ("item tag"), 11:w272) -> (3:w264:refnum<k9>)  [unwired: 4 in, 1 out]
        n156 = Set Menu Item Info(6:w261, 7:"Auto Scale Z" ("item tag"), 11:w264) -> (3:w259:refnum<k9>)  [unwired: 4 in, 1 out]
        n157 = Select(t="Hide Z Scale" ("item tag"), s=w249, f="Show Z Scale" ("item tag")) -> (s? t:f=w250:string)
        n158 = Set Menu Item Info(7:"Show Z Scale" ("item tag"), 10:w250, 11:w259) -> ()  [unwired: 4 in, 2 out]
        n159 = event-data("Discard?"=FALSE) -> ()  [unwired: 1 in, 1 out]
      }
      event "Channel 1", "Channel 2", "Channel 3", "Channel 4", "Channel 5", "Channel 6": Shortcut Menu Selection (User) {
        n160 = event-data() -> ("ItemPath"=w300:string, "ItemTag"=w301:string, "CtlRef"=w297:refnum<vi>)  [unwired: 1 in]
        n161 = Match Pattern(string=w300, regular expression=":") -> (before substring=w298:string, after substring=w294:string)  [unwired: 1 in, 2 out]
        n162 = case shown="\"Save Image\"" w298 {
          selector: w298 -> [_ _ w335 _ _ _ _ _ _ w431 _ _ _ _]
          tunnel: w297 -> [_ w315 w341 w366 _ w388 _ w402 w412 w429 w453 _ _ w462]
          tunnel: w301 -> [_ _ _ _ _ _ _ _ _ _ _ _ _ _]
          tunnel: w296 -> [_ w316 _ w369 w380 w390 _ w401 w413 w427 w449 _ _ _]
          tunnel: w295 -> [_ w314 _ w368 _ w389 _ _ _ _ _ _ _ _]
          tunnel: w294 -> [_ w303 _ _ _ _ _ _ _ _ _ _ _ _]
          frame Default {
          }
          frame "Color Map" {
            w309 = refnum<vi> refnum  # ImageControl
            w305 = u32 5 items=["Grayscale", "Binary", "Gradient", "Rainbow", "Temperature", "User Defined", "Binary 16 Bit", "Gradient 16 Bit", "Rainbow 16 Bit", "Temperature 16 Bit", "User Defined 16 Bit"] ("Palette:Palette Type")
            n163 = for {
              tunnel: w316 -> [w332] mode=indexing
              tunnel: [w333] -> w313
              tunnel: w315 -> [w331]
              i -> [w333]
              stop <- w330 stop-if-true
              n164 = Equal?(x=w331, y=w332) -> (x = y?=w330:bool)
            }
            n165 = Index Array(array=w314, index=w313) -> (element=w312:refnum<vi>)
            n166 = property class="Clust (strict)"(reference=w312) -> ("Controls[]"=w311:refnum<vi>[])  [unwired: 1 in, 2 out]
            n167 = property class="ImageControl"(reference=w315, "Palette Type"=w305) -> (reference out=w317:refnum<vi>)  [unwired: 1 in, 1 out]
            n168 = Index Array(array=w311, index=0) -> (element=w308:refnum<vi>)
            n169 = case shown="\"Glow\"" w303 {
              tunnel: [cluster{u8, u8, u8}[] [{0, 0, 0}, {1, 1, 1}, {2, 2, 2}, {3, 3, 3}, {4, 4, 4}, {5, 5, 5}, {6, 6, 6}, {7, 7, 7}, {8, 8, 8}, {9, 9, 9}, {10, 10, 10}, {11, 11, 11}, {12, 12, 12}, {13, 13, 13}, {14, 14, 14}, {15, 15, 15}, {16, 16, 16}, {17, 17, 17}, {18, 18, 18}, {19, 19, 19}, {20, 20, 20}, {21, 21, 21}, {22, 22, 22}, {23, 23, 23}, {24, 24, 24}, {25, 25, 25}, {26, 26, 26}, {27, 27, 27}, {28, 28, 28}, {29, 29, 29}, {30, 30, 30}, {31, 31, 31}, {32, 32, 32}, {33, 33, 33}, {34, 34, 34}, {35, 35, 35}, {36, 36, 36}, {37, 37, 37}, {38, 38, 38}, {39, 39, 39}, {40, 40, 40}, {41, 41, 41}, {42, 42, 42}, {43, 43, 43}, {44, 44, 44}, {45, 45, 45}, {46, 46, 46}, {47, 47, 47}, {48, 48, 48}, {49, 49, 49}, {50, 50, 50}, {51, 51, 51}, {52, 52, 52}, {53, 53, 53}, {54, 54, 54}, {55, 55, 55}, {56, 56, 56}, {57, 57, 57}, {58, 58, 58}, {59, 59, 59}, {60, 60, 60}, {61, 61, 61}, {62, 62, 62}, {63, 63, 63}, {64, 64, 64}, {65, 65, 65}, {66, 66, 66}, {67, 67, 67}, {68, 68, 68}, {69, 69, 69}, {70, 70, 70}, {71, 71, 71}, {72, 72, 72}, {73, 73, 73}, {74, 74, 74}, {75, 75, 75}, {76, 76, 76}, {77, 77, 77}, {78, 78, 78}, {79, 79, 79}, {80, 80, 80}, {81, 81, 81}, {82, 82, 82}, {83, 83, 83}, {84, 84, 84}, {85, 85, 85}, {86, 86, 86}, {87, 87, 87}, {88, 88, 88}, {89, 89, 89}, {90, 90, 90}, {91, 91, 91}, {92, 92, 92}, {93, 93, 93}, {94, 94, 94}, {95, 95, 95}, {96, 96, 96}, {97, 97, 97}, {98, 98, 98}, {99, 99, 99}, {100, 100, 100}, {101, 101, 101}, {102, 102, 102}, {103, 103, 103}, {104, 104, 104}, {105, 105, 105}, {106, 106, 106}, {107, 107, 107}, {108, 108, 108}, {109, 109, 109}, {110, 110, 110}, {111, 111, 111}, {112, 112, 112}, {113, 113, 113}, {114, 114, 114}, {115, 115, 115}, {116, 116, 116}, {117, 117, 117}, {118, 118, 118}, {119, 119, 119}, {120, 120, 120}, {121, 121, 121}, {122, 122, 122}, {123, 123, 123}, {124, 124, 124}, {125, 125, 125}, {126, 126, 126}, {127, 127, 127}, {128, 128, 128}, {129, 129, 129}, {130, 130, 130}, {131, 131, 131}, {132, 132, 132}, {133, 133, 133}, {134, 134, 134}, {135, 135, 135}, {136, 136, 136}, {137, 137, 137}, {138, 138, 138}, {139, 139, 139}, {140, 140, 140}, {141, 141, 141}, {142, 142, 142}, {143, 143, 143}, {144, 144, 144}, {145, 145, 145}, {146, 146, 146}, {147, 147, 147}, {148, 148, 148}, {149, 149, 149}, {150, 150, 150}, {151, 151, 151}, {152, 152, 152}, {153, 153, 153}, {154, 154, 154}, {155, 155, 155}, {156, 156, 156}, {157, 157, 157}, {158, 158, 158}, {159, 159, 159}, {160, 160, 160}, {161, 161, 161}, {162, 162, 162}, {163, 163, 163}, {164, 164, 164}, {165, 165, 165}, {166, 166, 166}, {167, 167, 167}, {168, 168, 168}, {169, 169, 169}, {170, 170, 170}, {171, 171, 171}, {172, 172, 172}, {173, 173, 173}, {174, 174, 174}, {175, 175, 175}, {176, 176, 176}, {177, 177, 177}, {178, 178, 178}, {179, 179, 179}, {180, 180, 180}, {181, 181, 181}, {182, 182, 182}, {183, 183, 183}, {184, 184, 184}, {185, 185, 185}, {186, 186, 186}, {187, 187, 187}, {188, 188, 188}, {189, 189, 189}, {190, 190, 190}, {191, 191, 191}, {192, 192, 192}, {193, 193, 193}, {194, 194, 194}, {195, 195, 195}, {196, 196, 196}, {197, 197, 197}, {198, 198, 198}, {199, 199, 199}, {200, 200, 200}, {201, 201, 201}, {202, 202, 202}, {203, 203, 203}, {204, 204, 204}, {205, 205, 205}, {206, 206, 206}, {207, 207, 207}, {208, 208, 208}, {209, 209, 209}, {210, 210, 210}, {211, 211, 211}, {212, 212, 212}, {213, 213, 213}, {214, 214, 214}, {215, 215, 215}, {216, 216, 216}, {217, 217, 217}, {218, 218, 218}, {219, 219, 219}, {220, 220, 220}, {221, 221, 221}, {222, 222, 222}, {223, 223, 223}, {224, 224, 224}, {225, 225, 225}, {226, 226, 226}, {227, 227, 227}, {228, 228, 228}, {229, 229, 229}, {230, 230, 230}, {231, 231, 231}, {232, 232, 232}, {233, 233, 233}, {234, 234, 234}, {235, 235, 235}, {236, 236, 236}, {237, 237, 237}, {238, 238, 238}, {239, 239, 239}, {240, 240, 240}, {241, 241, 241}, {242, 242, 242}, {243, 243, 243}, {244, 244, 244}, {245, 245, 245}, {246, 246, 246}, {247, 247, 247}, {248, 248, 248}, {249, 249, 249}, {250, 250, 250}, {251, 251, 251}, {252, 252, 252}, {253, 253, 253}, {254, 254, 254}, {255, 255, 255}] ("Array") cluster{u8, u8, u8}[] [{0, 0, 0}, {1, 0, 0}, {2, 0, 0}, {3, 0, 0}, {4, 0, 0}, {5, 0, 0}, {6, 0, 0}, {7, 0, 0}, {8, 0, 0}, {9, 0, 0}, {10, 0, 0}, {11, 0, 0}, {12, 0, 0}, {13, 0, 0}, {14, 0, 0}, {15, 0, 0}, {16, 0, 0}, {17, 0, 0}, {18, 0, 0}, {19, 0, 0}, {20, 0, 0}, {21, 0, 0}, {22, 0, 0}, {23, 0, 0}, {24, 0, 0}, {25, 0, 0}, {26, 0, 0}, {27, 0, 0}, {28, 0, 0}, {29, 0, 0}, {30, 0, 0}, {31, 0, 0}, {32, 0, 0}, {33, 0, 0}, {34, 0, 0}, {35, 0, 0}, {36, 0, 0}, {37, 0, 0}, {38, 0, 0}, {39, 0, 0}, {40, 0, 0}, {41, 0, 0}, {42, 0, 0}, {43, 0, 0}, {44, 0, 0}, {45, 0, 0}, {46, 0, 0}, {47, 0, 0}, {48, 0, 0}, {49, 0, 0}, {50, 0, 0}, {51, 0, 0}, {52, 0, 0}, {53, 0, 0}, {54, 0, 0}, {55, 0, 0}, {56, 0, 0}, {57, 0, 0}, {58, 0, 0}, {59, 0, 0}, {60, 0, 0}, {61, 0, 0}, {62, 0, 0}, {63, 0, 0}, {64, 0, 0}, {65, 0, 0}, {66, 0, 0}, {67, 0, 0}, {68, 0, 0}, {69, 0, 0}, {70, 0, 0}, {71, 0, 0}, {72, 0, 0}, {73, 0, 0}, {74, 0, 0}, {75, 0, 0}, {76, 0, 0}, {77, 0, 0}, {78, 0, 0}, {79, 0, 0}, {80, 0, 0}, {81, 0, 0}, {82, 0, 0}, {83, 0, 0}, {84, 0, 0}, {85, 0, 0}, {86, 0, 0}, {87, 0, 0}, {88, 0, 0}, {89, 0, 0}, {90, 0, 0}, {91, 0, 0}, {92, 0, 0}, {93, 0, 0}, {94, 0, 0}, {95, 0, 0}, {96, 0, 0}, {97, 0, 0}, {98, 0, 0}, {99, 0, 0}, {100, 0, 0}, {101, 0, 0}, {102, 0, 0}, {103, 0, 0}, {104, 0, 0}, {105, 0, 0}, {106, 0, 0}, {107, 0, 0}, {108, 0, 0}, {109, 0, 0}, {110, 0, 0}, {111, 0, 0}, {112, 0, 0}, {113, 0, 0}, {114, 0, 0}, {115, 0, 0}, {116, 0, 0}, {117, 0, 0}, {118, 0, 0}, {119, 0, 0}, {120, 0, 0}, {121, 0, 0}, {122, 0, 0}, {123, 0, 0}, {124, 0, 0}, {125, 0, 0}, {126, 0, 0}, {127, 0, 0}, {128, 0, 0}, {129, 0, 0}, {130, 0, 0}, {131, 0, 0}, {132, 0, 0}, {133, 0, 0}, {134, 0, 0}, {135, 0, 0}, {136, 0, 0}, {137, 0, 0}, {138, 0, 0}, {139, 0, 0}, {140, 0, 0}, {141, 0, 0}, {142, 0, 0}, {143, 0, 0}, {144, 0, 0}, {145, 0, 0}, {146, 0, 0}, {147, 0, 0}, {148, 0, 0}, {149, 0, 0}, {150, 0, 0}, {151, 0, 0}, {152, 0, 0}, {153, 0, 0}, {154, 0, 0}, {155, 0, 0}, {156, 0, 0}, {157, 0, 0}, {158, 0, 0}, {159, 0, 0}, {160, 0, 0}, {161, 0, 0}, {162, 0, 0}, {163, 0, 0}, {164, 0, 0}, {165, 0, 0}, {166, 0, 0}, {167, 0, 0}, {168, 0, 0}, {169, 0, 0}, {170, 0, 0}, {171, 0, 0}, {172, 0, 0}, {173, 0, 0}, {174, 0, 0}, {175, 0, 0}, {176, 0, 0}, {177, 0, 0}, {178, 0, 0}, {179, 0, 0}, {180, 0, 0}, {181, 0, 0}, {182, 0, 0}, {183, 0, 0}, {184, 0, 0}, {185, 0, 0}, {186, 0, 0}, {187, 0, 0}, {188, 0, 0}, {189, 0, 0}, {190, 0, 0}, {191, 0, 0}, {192, 0, 0}, {193, 0, 0}, {194, 0, 0}, {195, 0, 0}, {196, 0, 0}, {197, 0, 0}, {198, 0, 0}, {199, 0, 0}, {200, 0, 0}, {201, 0, 0}, {202, 0, 0}, {203, 0, 0}, {204, 0, 0}, {205, 0, 0}, {206, 0, 0}, {207, 0, 0}, {208, 0, 0}, {209, 0, 0}, {210, 0, 0}, {211, 0, 0}, {212, 0, 0}, {213, 0, 0}, {214, 0, 0}, {215, 0, 0}, {216, 0, 0}, {217, 0, 0}, {218, 0, 0}, {219, 0, 0}, {220, 0, 0}, {221, 0, 0}, {222, 0, 0}, {223, 0, 0}, {224, 0, 0}, {225, 0, 0}, {226, 0, 0}, {227, 0, 0}, {228, 0, 0}, {229, 0, 0}, {230, 0, 0}, {231, 0, 0}, {232, 0, 0}, {233, 0, 0}, {234, 0, 0}, {235, 0, 0}, {236, 0, 0}, {237, 0, 0}, {238, 0, 0}, {239, 0, 0}, {240, 0, 0}, {241, 0, 0}, {242, 0, 0}, {243, 0, 0}, {244, 0, 0}, {245, 0, 0}, {246, 0, 0}, {247, 0, 0}, {248, 0, 0}, {249, 0, 0}, {250, 0, 0}, {251, 0, 0}, {252, 0, 0}, {253, 0, 0}, {254, 0, 0}, {255, 0, 0}] ("Array") cluster{u8, u8, u8}[] [{0, 0, 0}, {0, 1, 0}, {0, 2, 0}, {0, 3, 0}, {0, 4, 0}, {0, 5, 0}, {0, 6, 0}, {0, 7, 0}, {0, 8, 0}, {0, 9, 0}, {0, 10, 0}, {0, 11, 0}, {0, 12, 0}, {0, 13, 0}, {0, 14, 0}, {0, 15, 0}, {0, 16, 0}, {0, 17, 0}, {0, 18, 0}, {0, 19, 0}, {0, 20, 0}, {0, 21, 0}, {0, 22, 0}, {0, 23, 0}, {0, 24, 0}, {0, 25, 0}, {0, 26, 0}, {0, 27, 0}, {0, 28, 0}, {0, 29, 0}, {0, 30, 0}, {0, 31, 0}, {0, 32, 0}, {0, 33, 0}, {0, 34, 0}, {0, 35, 0}, {0, 36, 0}, {0, 37, 0}, {0, 38, 0}, {0, 39, 0}, {0, 40, 0}, {0, 41, 0}, {0, 42, 0}, {0, 43, 0}, {0, 44, 0}, {0, 45, 0}, {0, 46, 0}, {0, 47, 0}, {0, 48, 0}, {0, 49, 0}, {0, 50, 0}, {0, 51, 0}, {0, 52, 0}, {0, 53, 0}, {0, 54, 0}, {0, 55, 0}, {0, 56, 0}, {0, 57, 0}, {0, 58, 0}, {0, 59, 0}, {0, 60, 0}, {0, 61, 0}, {0, 62, 0}, {0, 63, 0}, {0, 64, 0}, {0, 65, 0}, {0, 66, 0}, {0, 67, 0}, {0, 68, 0}, {0, 69, 0}, {0, 70, 0}, {0, 71, 0}, {0, 72, 0}, {0, 73, 0}, {0, 74, 0}, {0, 75, 0}, {0, 76, 0}, {0, 77, 0}, {0, 78, 0}, {0, 79, 0}, {0, 80, 0}, {0, 81, 0}, {0, 82, 0}, {0, 83, 0}, {0, 84, 0}, {0, 85, 0}, {0, 86, 0}, {0, 87, 0}, {0, 88, 0}, {0, 89, 0}, {0, 90, 0}, {0, 91, 0}, {0, 92, 0}, {0, 93, 0}, {0, 94, 0}, {0, 95, 0}, {0, 96, 0}, {0, 97, 0}, {0, 98, 0}, {0, 99, 0}, {0, 100, 0}, {0, 101, 0}, {0, 102, 0}, {0, 103, 0}, {0, 104, 0}, {0, 105, 0}, {0, 106, 0}, {0, 107, 0}, {0, 108, 0}, {0, 109, 0}, {0, 110, 0}, {0, 111, 0}, {0, 112, 0}, {0, 113, 0}, {0, 114, 0}, {0, 115, 0}, {0, 116, 0}, {0, 117, 0}, {0, 118, 0}, {0, 119, 0}, {0, 120, 0}, {0, 121, 0}, {0, 122, 0}, {0, 123, 0}, {0, 124, 0}, {0, 125, 0}, {0, 126, 0}, {0, 127, 0}, {0, 128, 0}, {0, 129, 0}, {0, 130, 0}, {0, 131, 0}, {0, 132, 0}, {0, 133, 0}, {0, 134, 0}, {0, 135, 0}, {0, 136, 0}, {0, 137, 0}, {0, 138, 0}, {0, 139, 0}, {0, 140, 0}, {0, 141, 0}, {0, 142, 0}, {0, 143, 0}, {0, 144, 0}, {0, 145, 0}, {0, 146, 0}, {0, 147, 0}, {0, 148, 0}, {0, 149, 0}, {0, 150, 0}, {0, 151, 0}, {0, 152, 0}, {0, 153, 0}, {0, 154, 0}, {0, 155, 0}, {0, 156, 0}, {0, 157, 0}, {0, 158, 0}, {0, 159, 0}, {0, 160, 0}, {0, 161, 0}, {0, 162, 0}, {0, 163, 0}, {0, 164, 0}, {0, 165, 0}, {0, 166, 0}, {0, 167, 0}, {0, 168, 0}, {0, 169, 0}, {0, 170, 0}, {0, 171, 0}, {0, 172, 0}, {0, 173, 0}, {0, 174, 0}, {0, 175, 0}, {0, 176, 0}, {0, 177, 0}, {0, 178, 0}, {0, 179, 0}, {0, 180, 0}, {0, 181, 0}, {0, 182, 0}, {0, 183, 0}, {0, 184, 0}, {0, 185, 0}, {0, 186, 0}, {0, 187, 0}, {0, 188, 0}, {0, 189, 0}, {0, 190, 0}, {0, 191, 0}, {0, 192, 0}, {0, 193, 0}, {0, 194, 0}, {0, 195, 0}, {0, 196, 0}, {0, 197, 0}, {0, 198, 0}, {0, 199, 0}, {0, 200, 0}, {0, 201, 0}, {0, 202, 0}, {0, 203, 0}, {0, 204, 0}, {0, 205, 0}, {0, 206, 0}, {0, 207, 0}, {0, 208, 0}, {0, 209, 0}, {0, 210, 0}, {0, 211, 0}, {0, 212, 0}, {0, 213, 0}, {0, 214, 0}, {0, 215, 0}, {0, 216, 0}, {0, 217, 0}, {0, 218, 0}, {0, 219, 0}, {0, 220, 0}, {0, 221, 0}, {0, 222, 0}, {0, 223, 0}, {0, 224, 0}, {0, 225, 0}, {0, 226, 0}, {0, 227, 0}, {0, 228, 0}, {0, 229, 0}, {0, 230, 0}, {0, 231, 0}, {0, 232, 0}, {0, 233, 0}, {0, 234, 0}, {0, 235, 0}, {0, 236, 0}, {0, 237, 0}, {0, 238, 0}, {0, 239, 0}, {0, 240, 0}, {0, 241, 0}, {0, 242, 0}, {0, 243, 0}, {0, 244, 0}, {0, 245, 0}, {0, 246, 0}, {0, 247, 0}, {0, 248, 0}, {0, 249, 0}, {0, 250, 0}, {0, 251, 0}, {0, 252, 0}, {0, 253, 0}, {0, 254, 0}, {0, 255, 0}] ("Array") cluster{u8, u8, u8}[] [{0, 0, 0}, {0, 0, 1}, {0, 0, 2}, {0, 0, 3}, {0, 0, 4}, {0, 0, 5}, {0, 0, 6}, {0, 0, 7}, {0, 0, 8}, {0, 0, 9}, {0, 0, 10}, {0, 0, 11}, {0, 0, 12}, {0, 0, 13}, {0, 0, 14}, {0, 0, 15}, {0, 0, 16}, {0, 0, 17}, {0, 0, 18}, {0, 0, 19}, {0, 0, 20}, {0, 0, 21}, {0, 0, 22}, {0, 0, 23}, {0, 0, 24}, {0, 0, 25}, {0, 0, 26}, {0, 0, 27}, {0, 0, 28}, {0, 0, 29}, {0, 0, 30}, {0, 0, 31}, {0, 0, 32}, {0, 0, 33}, {0, 0, 34}, {0, 0, 35}, {0, 0, 36}, {0, 0, 37}, {0, 0, 38}, {0, 0, 39}, {0, 0, 40}, {0, 0, 41}, {0, 0, 42}, {0, 0, 43}, {0, 0, 44}, {0, 0, 45}, {0, 0, 46}, {0, 0, 47}, {0, 0, 48}, {0, 0, 49}, {0, 0, 50}, {0, 0, 51}, {0, 0, 52}, {0, 0, 53}, {0, 0, 54}, {0, 0, 55}, {0, 0, 56}, {0, 0, 57}, {0, 0, 58}, {0, 0, 59}, {0, 0, 60}, {0, 0, 61}, {0, 0, 62}, {0, 0, 63}, {0, 0, 64}, {0, 0, 65}, {0, 0, 66}, {0, 0, 67}, {0, 0, 68}, {0, 0, 69}, {0, 0, 70}, {0, 0, 71}, {0, 0, 72}, {0, 0, 73}, {0, 0, 74}, {0, 0, 75}, {0, 0, 76}, {0, 0, 77}, {0, 0, 78}, {0, 0, 79}, {0, 0, 80}, {0, 0, 81}, {0, 0, 82}, {0, 0, 83}, {0, 0, 84}, {0, 0, 85}, {0, 0, 86}, {0, 0, 87}, {0, 0, 88}, {0, 0, 89}, {0, 0, 90}, {0, 0, 91}, {0, 0, 92}, {0, 0, 93}, {0, 0, 94}, {0, 0, 95}, {0, 0, 96}, {0, 0, 97}, {0, 0, 98}, {0, 0, 99}, {0, 0, 100}, {0, 0, 101}, {0, 0, 102}, {0, 0, 103}, {0, 0, 104}, {0, 0, 105}, {0, 0, 106}, {0, 0, 107}, {0, 0, 108}, {0, 0, 109}, {0, 0, 110}, {0, 0, 111}, {0, 0, 112}, {0, 0, 113}, {0, 0, 114}, {0, 0, 115}, {0, 0, 116}, {0, 0, 117}, {0, 0, 118}, {0, 0, 119}, {0, 0, 120}, {0, 0, 121}, {0, 0, 122}, {0, 0, 123}, {0, 0, 124}, {0, 0, 125}, {0, 0, 126}, {0, 0, 127}, {0, 0, 128}, {0, 0, 129}, {0, 0, 130}, {0, 0, 131}, {0, 0, 132}, {0, 0, 133}, {0, 0, 134}, {0, 0, 135}, {0, 0, 136}, {0, 0, 137}, {0, 0, 138}, {0, 0, 139}, {0, 0, 140}, {0, 0, 141}, {0, 0, 142}, {0, 0, 143}, {0, 0, 144}, {0, 0, 145}, {0, 0, 146}, {0, 0, 147}, {0, 0, 148}, {0, 0, 149}, {0, 0, 150}, {0, 0, 151}, {0, 0, 152}, {0, 0, 153}, {0, 0, 154}, {0, 0, 155}, {0, 0, 156}, {0, 0, 157}, {0, 0, 158}, {0, 0, 159}, {0, 0, 160}, {0, 0, 161}, {0, 0, 162}, {0, 0, 163}, {0, 0, 164}, {0, 0, 165}, {0, 0, 166}, {0, 0, 167}, {0, 0, 168}, {0, 0, 169}, {0, 0, 170}, {0, 0, 171}, {0, 0, 172}, {0, 0, 173}, {0, 0, 174}, {0, 0, 175}, {0, 0, 176}, {0, 0, 177}, {0, 0, 178}, {0, 0, 179}, {0, 0, 180}, {0, 0, 181}, {0, 0, 182}, {0, 0, 183}, {0, 0, 184}, {0, 0, 185}, {0, 0, 186}, {0, 0, 187}, {0, 0, 188}, {0, 0, 189}, {0, 0, 190}, {0, 0, 191}, {0, 0, 192}, {0, 0, 193}, {0, 0, 194}, {0, 0, 195}, {0, 0, 196}, {0, 0, 197}, {0, 0, 198}, {0, 0, 199}, {0, 0, 200}, {0, 0, 201}, {0, 0, 202}, {0, 0, 203}, {0, 0, 204}, {0, 0, 205}, {0, 0, 206}, {0, 0, 207}, {0, 0, 208}, {0, 0, 209}, {0, 0, 210}, {0, 0, 211}, {0, 0, 212}, {0, 0, 213}, {0, 0, 214}, {0, 0, 215}, {0, 0, 216}, {0, 0, 217}, {0, 0, 218}, {0, 0, 219}, {0, 0, 220}, {0, 0, 221}, {0, 0, 222}, {0, 0, 223}, {0, 0, 224}, {0, 0, 225}, {0, 0, 226}, {0, 0, 227}, {0, 0, 228}, {0, 0, 229}, {0, 0, 230}, {0, 0, 231}, {0, 0, 232}, {0, 0, 233}, {0, 0, 234}, {0, 0, 235}, {0, 0, 236}, {0, 0, 237}, {0, 0, 238}, {0, 0, 239}, {0, 0, 240}, {0, 0, 241}, {0, 0, 242}, {0, 0, 243}, {0, 0, 244}, {0, 0, 245}, {0, 0, 246}, {0, 0, 247}, {0, 0, 248}, {0, 0, 249}, {0, 0, 250}, {0, 0, 251}, {0, 0, 252}, {0, 0, 253}, {0, 0, 254}, {0, 0, 255}] ("Array") cluster{u8, u8, u8}[] [{0, 0, 0}, {0, 1, 1}, {0, 2, 2}, {0, 3, 3}, {0, 4, 4}, {0, 5, 5}, {0, 6, 6}, {0, 7, 7}, {0, 8, 8}, {0, 9, 9}, {0, 10, 10}, {0, 11, 11}, {0, 12, 12}, {0, 13, 13}, {0, 14, 14}, {0, 15, 15}, {0, 16, 16}, {0, 17, 17}, {0, 18, 18}, {0, 19, 19}, {0, 20, 20}, {0, 21, 21}, {0, 22, 22}, {0, 23, 23}, {0, 24, 24}, {0, 25, 25}, {0, 26, 26}, {0, 27, 27}, {0, 28, 28}, {0, 29, 29}, {0, 30, 30}, {0, 31, 31}, {0, 32, 32}, {0, 33, 33}, {0, 34, 34}, {0, 35, 35}, {0, 36, 36}, {0, 37, 37}, {0, 38, 38}, {0, 39, 39}, {0, 40, 40}, {0, 41, 41}, {0, 42, 42}, {0, 43, 43}, {0, 44, 44}, {0, 45, 45}, {0, 46, 46}, {0, 47, 47}, {0, 48, 48}, {0, 49, 49}, {0, 50, 50}, {0, 51, 51}, {0, 52, 52}, {0, 53, 53}, {0, 54, 54}, {0, 55, 55}, {0, 56, 56}, {0, 57, 57}, {0, 58, 58}, {0, 59, 59}, {0, 60, 60}, {0, 61, 61}, {0, 62, 62}, {0, 63, 63}, {0, 64, 64}, {0, 65, 65}, {0, 66, 66}, {0, 67, 67}, {0, 68, 68}, {0, 69, 69}, {0, 70, 70}, {0, 71, 71}, {0, 72, 72}, {0, 73, 73}, {0, 74, 74}, {0, 75, 75}, {0, 76, 76}, {0, 77, 77}, {0, 78, 78}, {0, 79, 79}, {0, 80, 80}, {0, 81, 81}, {0, 82, 82}, {0, 83, 83}, {0, 84, 84}, {0, 85, 85}, {0, 86, 86}, {0, 87, 87}, {0, 88, 88}, {0, 89, 89}, {0, 90, 90}, {0, 91, 91}, {0, 92, 92}, {0, 93, 93}, {0, 94, 94}, {0, 95, 95}, {0, 96, 96}, {0, 97, 97}, {0, 98, 98}, {0, 99, 99}, {0, 100, 100}, {0, 101, 101}, {0, 102, 102}, {0, 103, 103}, {0, 104, 104}, {0, 105, 105}, {0, 106, 106}, {0, 107, 107}, {0, 108, 108}, {0, 109, 109}, {0, 110, 110}, {0, 111, 111}, {0, 112, 112}, {0, 113, 113}, {0, 114, 114}, {0, 115, 115}, {0, 116, 116}, {0, 117, 117}, {0, 118, 118}, {0, 119, 119}, {0, 120, 120}, {0, 121, 121}, {0, 122, 122}, {0, 123, 123}, {0, 124, 124}, {0, 125, 125}, {0, 126, 126}, {0, 127, 127}, {0, 128, 128}, {0, 129, 129}, {0, 130, 130}, {0, 131, 131}, {0, 132, 132}, {0, 133, 133}, {0, 134, 134}, {0, 135, 135}, {0, 136, 136}, {0, 137, 137}, {0, 138, 138}, {0, 139, 139}, {0, 140, 140}, {0, 141, 141}, {0, 142, 142}, {0, 143, 143}, {0, 144, 144}, {0, 145, 145}, {0, 146, 146}, {0, 147, 147}, {0, 148, 148}, {0, 149, 149}, {0, 150, 150}, {0, 151, 151}, {0, 152, 152}, {0, 153, 153}, {0, 154, 154}, {0, 155, 155}, {0, 156, 156}, {0, 157, 157}, {0, 158, 158}, {0, 159, 159}, {0, 160, 160}, {0, 161, 161}, {0, 162, 162}, {0, 163, 163}, {0, 164, 164}, {0, 165, 165}, {0, 166, 166}, {0, 167, 167}, {0, 168, 168}, {0, 169, 169}, {0, 170, 170}, {0, 171, 171}, {0, 172, 172}, {0, 173, 173}, {0, 174, 174}, {0, 175, 175}, {0, 176, 176}, {0, 177, 177}, {0, 178, 178}, {0, 179, 179}, {0, 180, 180}, {0, 181, 181}, {0, 182, 182}, {0, 183, 183}, {0, 184, 184}, {0, 185, 185}, {0, 186, 186}, {0, 187, 187}, {0, 188, 188}, {0, 189, 189}, {0, 190, 190}, {0, 191, 191}, {0, 192, 192}, {0, 193, 193}, {0, 194, 194}, {0, 195, 195}, {0, 196, 196}, {0, 197, 197}, {0, 198, 198}, {0, 199, 199}, {0, 200, 200}, {0, 201, 201}, {0, 202, 202}, {0, 203, 203}, {0, 204, 204}, {0, 205, 205}, {0, 206, 206}, {0, 207, 207}, {0, 208, 208}, {0, 209, 209}, {0, 210, 210}, {0, 211, 211}, {0, 212, 212}, {0, 213, 213}, {0, 214, 214}, {0, 215, 215}, {0, 216, 216}, {0, 217, 217}, {0, 218, 218}, {0, 219, 219}, {0, 220, 220}, {0, 221, 221}, {0, 222, 222}, {0, 223, 223}, {0, 224, 224}, {0, 225, 225}, {0, 226, 226}, {0, 227, 227}, {0, 228, 228}, {0, 229, 229}, {0, 230, 230}, {0, 231, 231}, {0, 232, 232}, {0, 233, 233}, {0, 234, 234}, {0, 235, 235}, {0, 236, 236}, {0, 237, 237}, {0, 238, 238}, {0, 239, 239}, {0, 240, 240}, {0, 241, 241}, {0, 242, 242}, {0, 243, 243}, {0, 244, 244}, {0, 245, 245}, {0, 246, 246}, {0, 247, 247}, {0, 248, 248}, {0, 249, 249}, {0, 250, 250}, {0, 251, 251}, {0, 252, 252}, {0, 253, 253}, {0, 254, 254}, {0, 255, 255}] ("Array") cluster{u8, u8, u8}[] [{0, 0, 0}, {1, 0, 1}, {2, 0, 2}, {3, 0, 3}, {4, 0, 4}, {5, 0, 5}, {6, 0, 6}, {7, 0, 7}, {8, 0, 8}, {9, 0, 9}, {10, 0, 10}, {11, 0, 11}, {12, 0, 12}, {13, 0, 13}, {14, 0, 14}, {15, 0, 15}, {16, 0, 16}, {17, 0, 17}, {18, 0, 18}, {19, 0, 19}, {20, 0, 20}, {21, 0, 21}, {22, 0, 22}, {23, 0, 23}, {24, 0, 24}, {25, 0, 25}, {26, 0, 26}, {27, 0, 27}, {28, 0, 28}, {29, 0, 29}, {30, 0, 30}, {31, 0, 31}, {32, 0, 32}, {33, 0, 33}, {34, 0, 34}, {35, 0, 35}, {36, 0, 36}, {37, 0, 37}, {38, 0, 38}, {39, 0, 39}, {40, 0, 40}, {41, 0, 41}, {42, 0, 42}, {43, 0, 43}, {44, 0, 44}, {45, 0, 45}, {46, 0, 46}, {47, 0, 47}, {48, 0, 48}, {49, 0, 49}, {50, 0, 50}, {51, 0, 51}, {52, 0, 52}, {53, 0, 53}, {54, 0, 54}, {55, 0, 55}, {56, 0, 56}, {57, 0, 57}, {58, 0, 58}, {59, 0, 59}, {60, 0, 60}, {61, 0, 61}, {62, 0, 62}, {63, 0, 63}, {64, 0, 64}, {65, 0, 65}, {66, 0, 66}, {67, 0, 67}, {68, 0, 68}, {69, 0, 69}, {70, 0, 70}, {71, 0, 71}, {72, 0, 72}, {73, 0, 73}, {74, 0, 74}, {75, 0, 75}, {76, 0, 76}, {77, 0, 77}, {78, 0, 78}, {79, 0, 79}, {80, 0, 80}, {81, 0, 81}, {82, 0, 82}, {83, 0, 83}, {84, 0, 84}, {85, 0, 85}, {86, 0, 86}, {87, 0, 87}, {88, 0, 88}, {89, 0, 89}, {90, 0, 90}, {91, 0, 91}, {92, 0, 92}, {93, 0, 93}, {94, 0, 94}, {95, 0, 95}, {96, 0, 96}, {97, 0, 97}, {98, 0, 98}, {99, 0, 99}, {100, 0, 100}, {101, 0, 101}, {102, 0, 102}, {103, 0, 103}, {104, 0, 104}, {105, 0, 105}, {106, 0, 106}, {107, 0, 107}, {108, 0, 108}, {109, 0, 109}, {110, 0, 110}, {111, 0, 111}, {112, 0, 112}, {113, 0, 113}, {114, 0, 114}, {115, 0, 115}, {116, 0, 116}, {117, 0, 117}, {118, 0, 118}, {119, 0, 119}, {120, 0, 120}, {121, 0, 121}, {122, 0, 122}, {123, 0, 123}, {124, 0, 124}, {125, 0, 125}, {126, 0, 126}, {127, 0, 127}, {128, 0, 128}, {129, 0, 129}, {130, 0, 130}, {131, 0, 131}, {132, 0, 132}, {133, 0, 133}, {134, 0, 134}, {135, 0, 135}, {136, 0, 136}, {137, 0, 137}, {138, 0, 138}, {139, 0, 139}, {140, 0, 140}, {141, 0, 141}, {142, 0, 142}, {143, 0, 143}, {144, 0, 144}, {145, 0, 145}, {146, 0, 146}, {147, 0, 147}, {148, 0, 148}, {149, 0, 149}, {150, 0, 150}, {151, 0, 151}, {152, 0, 152}, {153, 0, 153}, {154, 0, 154}, {155, 0, 155}, {156, 0, 156}, {157, 0, 157}, {158, 0, 158}, {159, 0, 159}, {160, 0, 160}, {161, 0, 161}, {162, 0, 162}, {163, 0, 163}, {164, 0, 164}, {165, 0, 165}, {166, 0, 166}, {167, 0, 167}, {168, 0, 168}, {169, 0, 169}, {170, 0, 170}, {171, 0, 171}, {172, 0, 172}, {173, 0, 173}, {174, 0, 174}, {175, 0, 175}, {176, 0, 176}, {177, 0, 177}, {178, 0, 178}, {179, 0, 179}, {180, 0, 180}, {181, 0, 181}, {182, 0, 182}, {183, 0, 183}, {184, 0, 184}, {185, 0, 185}, {186, 0, 186}, {187, 0, 187}, {188, 0, 188}, {189, 0, 189}, {190, 0, 190}, {191, 0, 191}, {192, 0, 192}, {193, 0, 193}, {194, 0, 194}, {195, 0, 195}, {196, 0, 196}, {197, 0, 197}, {198, 0, 198}, {199, 0, 199}, {200, 0, 200}, {201, 0, 201}, {202, 0, 202}, {203, 0, 203}, {204, 0, 204}, {205, 0, 205}, {206, 0, 206}, {207, 0, 207}, {208, 0, 208}, {209, 0, 209}, {210, 0, 210}, {211, 0, 211}, {212, 0, 212}, {213, 0, 213}, {214, 0, 214}, {215, 0, 215}, {216, 0, 216}, {217, 0, 217}, {218, 0, 218}, {219, 0, 219}, {220, 0, 220}, {221, 0, 221}, {222, 0, 222}, {223, 0, 223}, {224, 0, 224}, {225, 0, 225}, {226, 0, 226}, {227, 0, 227}, {228, 0, 228}, {229, 0, 229}, {230, 0, 230}, {231, 0, 231}, {232, 0, 232}, {233, 0, 233}, {234, 0, 234}, {235, 0, 235}, {236, 0, 236}, {237, 0, 237}, {238, 0, 238}, {239, 0, 239}, {240, 0, 240}, {241, 0, 241}, {242, 0, 242}, {243, 0, 243}, {244, 0, 244}, {245, 0, 245}, {246, 0, 246}, {247, 0, 247}, {248, 0, 248}, {249, 0, 249}, {250, 0, 250}, {251, 0, 251}, {252, 0, 252}, {253, 0, 253}, {254, 0, 254}, {255, 0, 255}] ("Array") cluster{u8, u8, u8}[] [{0, 0, 0}, {1, 1, 0}, {2, 2, 0}, {3, 3, 0}, {4, 4, 0}, {5, 5, 0}, {6, 6, 0}, {7, 7, 0}, {8, 8, 0}, {9, 9, 0}, {10, 10, 0}, {11, 11, 0}, {12, 12, 0}, {13, 13, 0}, {14, 14, 0}, {15, 15, 0}, {16, 16, 0}, {17, 17, 0}, {18, 18, 0}, {19, 19, 0}, {20, 20, 0}, {21, 21, 0}, {22, 22, 0}, {23, 23, 0}, {24, 24, 0}, {25, 25, 0}, {26, 26, 0}, {27, 27, 0}, {28, 28, 0}, {29, 29, 0}, {30, 30, 0}, {31, 31, 0}, {32, 32, 0}, {33, 33, 0}, {34, 34, 0}, {35, 35, 0}, {36, 36, 0}, {37, 37, 0}, {38, 38, 0}, {39, 39, 0}, {40, 40, 0}, {41, 41, 0}, {42, 42, 0}, {43, 43, 0}, {44, 44, 0}, {45, 45, 0}, {46, 46, 0}, {47, 47, 0}, {48, 48, 0}, {49, 49, 0}, {50, 50, 0}, {51, 51, 0}, {52, 52, 0}, {53, 53, 0}, {54, 54, 0}, {55, 55, 0}, {56, 56, 0}, {57, 57, 0}, {58, 58, 0}, {59, 59, 0}, {60, 60, 0}, {61, 61, 0}, {62, 62, 0}, {63, 63, 0}, {64, 64, 0}, {65, 65, 0}, {66, 66, 0}, {67, 67, 0}, {68, 68, 0}, {69, 69, 0}, {70, 70, 0}, {71, 71, 0}, {72, 72, 0}, {73, 73, 0}, {74, 74, 0}, {75, 75, 0}, {76, 76, 0}, {77, 77, 0}, {78, 78, 0}, {79, 79, 0}, {80, 80, 0}, {81, 81, 0}, {82, 82, 0}, {83, 83, 0}, {84, 84, 0}, {85, 85, 0}, {86, 86, 0}, {87, 87, 0}, {88, 88, 0}, {89, 89, 0}, {90, 90, 0}, {91, 91, 0}, {92, 92, 0}, {93, 93, 0}, {94, 94, 0}, {95, 95, 0}, {96, 96, 0}, {97, 97, 0}, {98, 98, 0}, {99, 99, 0}, {100, 100, 0}, {101, 101, 0}, {102, 102, 0}, {103, 103, 0}, {104, 104, 0}, {105, 105, 0}, {106, 106, 0}, {107, 107, 0}, {108, 108, 0}, {109, 109, 0}, {110, 110, 0}, {111, 111, 0}, {112, 112, 0}, {113, 113, 0}, {114, 114, 0}, {115, 115, 0}, {116, 116, 0}, {117, 117, 0}, {118, 118, 0}, {119, 119, 0}, {120, 120, 0}, {121, 121, 0}, {122, 122, 0}, {123, 123, 0}, {124, 124, 0}, {125, 125, 0}, {126, 126, 0}, {127, 127, 0}, {128, 128, 0}, {129, 129, 0}, {130, 130, 0}, {131, 131, 0}, {132, 132, 0}, {133, 133, 0}, {134, 134, 0}, {135, 135, 0}, {136, 136, 0}, {137, 137, 0}, {138, 138, 0}, {139, 139, 0}, {140, 140, 0}, {141, 141, 0}, {142, 142, 0}, {143, 143, 0}, {144, 144, 0}, {145, 145, 0}, {146, 146, 0}, {147, 147, 0}, {148, 148, 0}, {149, 149, 0}, {150, 150, 0}, {151, 151, 0}, {152, 152, 0}, {153, 153, 0}, {154, 154, 0}, {155, 155, 0}, {156, 156, 0}, {157, 157, 0}, {158, 158, 0}, {159, 159, 0}, {160, 160, 0}, {161, 161, 0}, {162, 162, 0}, {163, 163, 0}, {164, 164, 0}, {165, 165, 0}, {166, 166, 0}, {167, 167, 0}, {168, 168, 0}, {169, 169, 0}, {170, 170, 0}, {171, 171, 0}, {172, 172, 0}, {173, 173, 0}, {174, 174, 0}, {175, 175, 0}, {176, 176, 0}, {177, 177, 0}, {178, 178, 0}, {179, 179, 0}, {180, 180, 0}, {181, 181, 0}, {182, 182, 0}, {183, 183, 0}, {184, 184, 0}, {185, 185, 0}, {186, 186, 0}, {187, 187, 0}, {188, 188, 0}, {189, 189, 0}, {190, 190, 0}, {191, 191, 0}, {192, 192, 0}, {193, 193, 0}, {194, 194, 0}, {195, 195, 0}, {196, 196, 0}, {197, 197, 0}, {198, 198, 0}, {199, 199, 0}, {200, 200, 0}, {201, 201, 0}, {202, 202, 0}, {203, 203, 0}, {204, 204, 0}, {205, 205, 0}, {206, 206, 0}, {207, 207, 0}, {208, 208, 0}, {209, 209, 0}, {210, 210, 0}, {211, 211, 0}, {212, 212, 0}, {213, 213, 0}, {214, 214, 0}, {215, 215, 0}, {216, 216, 0}, {217, 217, 0}, {218, 218, 0}, {219, 219, 0}, {220, 220, 0}, {221, 221, 0}, {222, 222, 0}, {223, 223, 0}, {224, 224, 0}, {225, 225, 0}, {226, 226, 0}, {227, 227, 0}, {228, 228, 0}, {229, 229, 0}, {230, 230, 0}, {231, 231, 0}, {232, 232, 0}, {233, 233, 0}, {234, 234, 0}, {235, 235, 0}, {236, 236, 0}, {237, 237, 0}, {238, 238, 0}, {239, 239, 0}, {240, 240, 0}, {241, 241, 0}, {242, 242, 0}, {243, 243, 0}, {244, 244, 0}, {245, 245, 0}, {246, 246, 0}, {247, 247, 0}, {248, 248, 0}, {249, 249, 0}, {250, 250, 0}, {251, 251, 0}, {252, 252, 0}, {253, 253, 0}, {254, 254, 0}, {255, 255, 0}] ("Array") cluster{u8, u8, u8}[] [{0, 0, 0}, {2, 0, 0}, {3, 0, 0}, {4, 0, 0}, {6, 0, 0}, {8, 0, 0}, {9, 0, 0}, {10, 0, 0}, {12, 0, 0}, {14, 0, 0}, {15, 0, 0}, {16, 0, 0}, {18, 0, 0}, {20, 0, 0}, {21, 0, 0}, {22, 0, 0}, {24, 0, 0}, {26, 0, 0}, {27, 0, 0}, {28, 0, 0}, {30, 0, 0}, {32, 0, 0}, {33, 0, 0}, {34, 0, 0}, {36, 0, 0}, {38, 0, 0}, {39, 0, 0}, {40, 0, 0}, {42, 0, 0}, {44, 0, 0}, {45, 0, 0}, {46, 0, 0}, {48, 0, 0}, {50, 0, 0}, {51, 0, 0}, {52, 0, 0}, {54, 0, 0}, {56, 0, 0}, {57, 0, 0}, {58, 0, 0}, {60, 0, 0}, {62, 0, 0}, {63, 0, 0}, {64, 0, 0}, {66, 0, 0}, {68, 0, 0}, {69, 0, 0}, {70, 0, 0}, {72, 0, 0}, {74, 0, 0}, {75, 0, 0}, {76, 0, 0}, {78, 0, 0}, {80, 0, 0}, {81, 0, 0}, {82, 0, 0}, {84, 0, 0}, {86, 0, 0}, {87, 0, 0}, {88, 0, 0}, {90, 0, 0}, {92, 0, 0}, {93, 0, 0}, {94, 0, 0}, {96, 0, 0}, {98, 0, 0}, {99, 0, 0}, {100, 0, 0}, {102, 0, 0}, {104, 0, 0}, {105, 0, 0}, {106, 0, 0}, {108, 0, 0}, {110, 0, 0}, {111, 0, 0}, {112, 0, 0}, {114, 0, 0}, {116, 0, 0}, {117, 0, 0}, {118, 0, 0}, {120, 0, 0}, {122, 0, 0}, {123, 0, 0}, {124, 0, 0}, {126, 0, 0}, {128, 0, 0}, {129, 0, 0}, {130, 0, 0}, {132, 0, 0}, {134, 0, 0}, {135, 0, 0}, {136, 0, 0}, {138, 0, 0}, {140, 0, 0}, {141, 0, 0}, {142, 0, 0}, {144, 0, 0}, {146, 0, 0}, {147, 0, 0}, {148, 0, 0}, {150, 0, 0}, {152, 0, 0}, {153, 0, 0}, {154, 0, 0}, {156, 0, 0}, {158, 0, 0}, {159, 0, 0}, {160, 0, 0}, {162, 0, 0}, {164, 0, 0}, {165, 0, 0}, {166, 0, 0}, {168, 0, 0}, {170, 0, 0}, {171, 0, 0}, {172, 0, 0}, {174, 0, 0}, {176, 0, 0}, {177, 0, 0}, {178, 0, 0}, {180, 0, 0}, {182, 0, 0}, {183, 0, 0}, {184, 0, 0}, {186, 0, 0}, {188, 0, 0}, {189, 0, 0}, {190, 0, 0}, {192, 0, 0}, {194, 0, 0}, {195, 0, 0}, {196, 0, 0}, {198, 0, 0}, {200, 0, 0}, {201, 0, 0}, {202, 0, 0}, {204, 0, 0}, {206, 0, 0}, {207, 0, 0}, {208, 0, 0}, {210, 0, 0}, {212, 0, 0}, {213, 0, 0}, {214, 0, 0}, {216, 0, 0}, {218, 0, 0}, {219, 0, 0}, {220, 0, 0}, {222, 0, 0}, {224, 0, 0}, {225, 0, 0}, {226, 0, 0}, {228, 0, 0}, {230, 0, 0}, {231, 0, 0}, {232, 0, 0}, {234, 0, 0}, {236, 0, 0}, {237, 0, 0}, {238, 0, 0}, {240, 0, 0}, {242, 0, 0}, {243, 0, 0}, {244, 0, 0}, {246, 0, 0}, {248, 0, 0}, {249, 0, 0}, {250, 0, 0}, {252, 0, 0}, {254, 0, 0}, {255, 0, 0}, {255, 3, 3}, {255, 7, 6}, {255, 10, 9}, {255, 14, 12}, {255, 17, 15}, {255, 20, 18}, {255, 24, 21}, {255, 27, 24}, {255, 31, 27}, {255, 34, 30}, {255, 37, 33}, {255, 41, 36}, {255, 44, 39}, {255, 48, 42}, {255, 51, 45}, {255, 54, 48}, {255, 58, 51}, {255, 61, 54}, {255, 65, 57}, {255, 68, 60}, {255, 71, 63}, {255, 75, 66}, {255, 78, 69}, {255, 82, 72}, {255, 85, 75}, {255, 88, 78}, {255, 92, 81}, {255, 95, 84}, {255, 99, 87}, {255, 102, 90}, {255, 105, 93}, {255, 109, 96}, {255, 112, 99}, {255, 116, 102}, {255, 119, 105}, {255, 122, 108}, {255, 126, 111}, {255, 129, 113}, {255, 133, 116}, {255, 136, 119}, {255, 139, 122}, {255, 143, 125}, {255, 146, 128}, {255, 150, 131}, {255, 153, 134}, {255, 156, 137}, {255, 160, 140}, {255, 163, 143}, {255, 167, 146}, {255, 170, 149}, {255, 173, 152}, {255, 177, 155}, {255, 180, 158}, {255, 184, 161}, {255, 187, 164}, {255, 190, 167}, {255, 194, 170}, {255, 197, 173}, {255, 201, 176}, {255, 204, 179}, {255, 207, 182}, {255, 211, 185}, {255, 214, 188}, {255, 218, 191}, {255, 221, 194}, {255, 224, 197}, {255, 228, 200}, {255, 231, 203}, {255, 235, 206}, {255, 238, 209}, {255, 241, 212}, {255, 245, 215}, {255, 248, 218}, {255, 252, 221}, {255, 255, 224}, {255, 255, 227}, {255, 255, 230}, {255, 255, 234}, {255, 255, 237}, {255, 255, 240}, {254, 254, 242}, {253, 253, 244}, {252, 252, 246}, {251, 251, 248}, {250, 250, 250}] ("Array 2") cluster{u8, u8, u8}[] [{0, 0, 0}, {0, 2, 0}, {0, 3, 0}, {0, 4, 0}, {0, 6, 0}, {0, 8, 0}, {0, 9, 0}, {0, 10, 0}, {0, 12, 0}, {0, 14, 0}, {0, 15, 0}, {0, 16, 0}, {0, 18, 0}, {0, 20, 0}, {0, 21, 0}, {0, 22, 0}, {0, 24, 0}, {0, 26, 0}, {0, 27, 0}, {0, 28, 0}, {0, 30, 0}, {0, 32, 0}, {0, 33, 0}, {0, 34, 0}, {0, 36, 0}, {0, 38, 0}, {0, 39, 0}, {0, 40, 0}, {0, 42, 0}, {0, 44, 0}, {0, 45, 0}, {0, 46, 0}, {0, 48, 0}, {0, 50, 0}, {0, 51, 0}, {0, 52, 0}, {0, 54, 0}, {0, 56, 0}, {0, 57, 0}, {0, 58, 0}, {0, 60, 0}, {0, 62, 0}, {0, 63, 0}, {0, 64, 0}, {0, 66, 0}, {0, 68, 0}, {0, 69, 0}, {0, 70, 0}, {0, 72, 0}, {0, 74, 0}, {0, 75, 0}, {0, 76, 0}, {0, 78, 0}, {0, 80, 0}, {0, 81, 0}, {0, 82, 0}, {0, 84, 0}, {0, 86, 0}, {0, 87, 0}, {0, 88, 0}, {0, 90, 0}, {0, 92, 0}, {0, 93, 0}, {0, 94, 0}, {0, 96, 0}, {0, 98, 0}, {0, 99, 0}, {0, 100, 0}, {0, 102, 0}, {0, 104, 0}, {0, 105, 0}, {0, 106, 0}, {0, 108, 0}, {0, 110, 0}, {0, 111, 0}, {0, 112, 0}, {0, 114, 0}, {0, 116, 0}, {0, 117, 0}, {0, 118, 0}, {0, 120, 0}, {0, 122, 0}, {0, 123, 0}, {0, 124, 0}, {0, 126, 0}, {0, 128, 0}, {0, 129, 0}, {0, 130, 0}, {0, 132, 0}, {0, 134, 0}, {0, 135, 0}, {0, 136, 0}, {0, 138, 0}, {0, 140, 0}, {0, 141, 0}, {0, 142, 0}, {0, 144, 0}, {0, 146, 0}, {0, 147, 0}, {0, 148, 0}, {0, 150, 0}, {0, 152, 0}, {0, 153, 0}, {0, 154, 0}, {0, 156, 0}, {0, 158, 0}, {0, 159, 0}, {0, 160, 0}, {0, 162, 0}, {0, 164, 0}, {0, 165, 0}, {0, 166, 0}, {0, 168, 0}, {0, 170, 0}, {0, 171, 0}, {0, 172, 0}, {0, 174, 0}, {0, 176, 0}, {0, 177, 0}, {0, 178, 0}, {0, 180, 0}, {0, 182, 0}, {0, 183, 0}, {0, 184, 0}, {0, 186, 0}, {0, 188, 0}, {0, 189, 0}, {0, 190, 0}, {0, 192, 0}, {0, 194, 0}, {0, 195, 0}, {0, 196, 0}, {0, 198, 0}, {0, 200, 0}, {0, 201, 0}, {0, 202, 0}, {0, 204, 0}, {0, 206, 0}, {0, 207, 0}, {0, 208, 0}, {0, 210, 0}, {0, 212, 0}, {0, 213, 0}, {0, 214, 0}, {0, 216, 0}, {0, 218, 0}, {0, 219, 0}, {0, 220, 0}, {0, 222, 0}, {0, 224, 0}, {0, 225, 0}, {0, 226, 0}, {0, 228, 0}, {0, 230, 0}, {0, 231, 0}, {0, 232, 0}, {0, 234, 0}, {0, 236, 0}, {0, 237, 0}, {0, 238, 0}, {0, 240, 0}, {0, 242, 0}, {0, 243, 0}, {0, 244, 0}, {0, 246, 0}, {0, 248, 0}, {0, 249, 0}, {0, 250, 0}, {0, 252, 0}, {0, 254, 0}, {0, 255, 0}, {3, 255, 3}, {7, 255, 6}, {10, 255, 9}, {14, 255, 12}, {17, 255, 15}, {20, 255, 18}, {24, 255, 21}, {27, 255, 24}, {31, 255, 27}, {34, 255, 30}, {37, 255, 33}, {41, 255, 36}, {44, 255, 39}, {48, 255, 42}, {51, 255, 45}, {54, 255, 48}, {58, 255, 51}, {61, 255, 54}, {65, 255, 57}, {68, 255, 60}, {71, 255, 63}, {75, 255, 66}, {78, 255, 69}, {82, 255, 72}, {85, 255, 75}, {88, 255, 78}, {92, 255, 81}, {95, 255, 84}, {99, 255, 87}, {102, 255, 90}, {105, 255, 93}, {109, 255, 96}, {112, 255, 99}, {116, 255, 102}, {119, 255, 105}, {122, 255, 108}, {126, 255, 111}, {129, 255, 113}, {133, 255, 116}, {136, 255, 119}, {139, 255, 122}, {143, 255, 125}, {146, 255, 128}, {150, 255, 131}, {153, 255, 134}, {156, 255, 137}, {160, 255, 140}, {163, 255, 143}, {167, 255, 146}, {170, 255, 149}, {173, 255, 152}, {177, 255, 155}, {180, 255, 158}, {184, 255, 161}, {187, 255, 164}, {190, 255, 167}, {194, 255, 170}, {197, 255, 173}, {201, 255, 176}, {204, 255, 179}, {207, 255, 182}, {211, 255, 185}, {214, 255, 188}, {218, 255, 191}, {221, 255, 194}, {224, 255, 197}, {228, 255, 200}, {231, 255, 203}, {235, 255, 206}, {238, 255, 209}, {241, 255, 212}, {245, 255, 215}, {248, 255, 218}, {252, 255, 221}, {255, 255, 224}, {255, 255, 227}, {255, 255, 230}, {255, 255, 234}, {255, 255, 237}, {255, 255, 240}, {254, 254, 242}, {253, 253, 244}, {252, 252, 246}, {251, 251, 248}, {250, 250, 250}] ("Array 2") cluster{u8, u8, u8}[] [{0, 0, 0}, {0, 0, 2}, {0, 0, 3}, {0, 0, 4}, {0, 0, 6}, {0, 0, 8}, {0, 0, 9}, {0, 0, 10}, {0, 0, 12}, {0, 0, 14}, {0, 0, 15}, {0, 0, 16}, {0, 0, 18}, {0, 0, 20}, {0, 0, 21}, {0, 0, 22}, {0, 0, 24}, {0, 0, 26}, {0, 0, 27}, {0, 0, 28}, {0, 0, 30}, {0, 0, 32}, {0, 0, 33}, {0, 0, 34}, {0, 0, 36}, {0, 0, 38}, {0, 0, 39}, {0, 0, 40}, {0, 0, 42}, {0, 0, 44}, {0, 0, 45}, {0, 0, 46}, {0, 0, 48}, {0, 0, 50}, {0, 0, 51}, {0, 0, 52}, {0, 0, 54}, {0, 0, 56}, {0, 0, 57}, {0, 0, 58}, {0, 0, 60}, {0, 0, 62}, {0, 0, 63}, {0, 0, 64}, {0, 0, 66}, {0, 0, 68}, {0, 0, 69}, {0, 0, 70}, {0, 0, 72}, {0, 0, 74}, {0, 0, 75}, {0, 0, 76}, {0, 0, 78}, {0, 0, 80}, {0, 0, 81}, {0, 0, 82}, {0, 0, 84}, {0, 0, 86}, {0, 0, 87}, {0, 0, 88}, {0, 0, 90}, {0, 0, 92}, {0, 0, 93}, {0, 0, 94}, {0, 0, 96}, {0, 0, 98}, {0, 0, 99}, {0, 0, 100}, {0, 0, 102}, {0, 0, 104}, {0, 0, 105}, {0, 0, 106}, {0, 0, 108}, {0, 0, 110}, {0, 0, 111}, {0, 0, 112}, {0, 0, 114}, {0, 0, 116}, {0, 0, 117}, {0, 0, 118}, {0, 0, 120}, {0, 0, 122}, {0, 0, 123}, {0, 0, 124}, {0, 0, 126}, {0, 0, 128}, {0, 0, 129}, {0, 0, 130}, {0, 0, 132}, {0, 0, 134}, {0, 0, 135}, {0, 0, 136}, {0, 0, 138}, {0, 0, 140}, {0, 0, 141}, {0, 0, 142}, {0, 0, 144}, {0, 0, 146}, {0, 0, 147}, {0, 0, 148}, {0, 0, 150}, {0, 0, 152}, {0, 0, 153}, {0, 0, 154}, {0, 0, 156}, {0, 0, 158}, {0, 0, 159}, {0, 0, 160}, {0, 0, 162}, {0, 0, 164}, {0, 0, 165}, {0, 0, 166}, {0, 0, 168}, {0, 0, 170}, {0, 0, 171}, {0, 0, 172}, {0, 0, 174}, {0, 0, 176}, {0, 0, 177}, {0, 0, 178}, {0, 0, 180}, {0, 0, 182}, {0, 0, 183}, {0, 0, 184}, {0, 0, 186}, {0, 0, 188}, {0, 0, 189}, {0, 0, 190}, {0, 0, 192}, {0, 0, 194}, {0, 0, 195}, {0, 0, 196}, {0, 0, 198}, {0, 0, 200}, {0, 0, 201}, {0, 0, 202}, {0, 0, 204}, {0, 0, 206}, {0, 0, 207}, {0, 0, 208}, {0, 0, 210}, {0, 0, 212}, {0, 0, 213}, {0, 0, 214}, {0, 0, 216}, {0, 0, 218}, {0, 0, 219}, {0, 0, 220}, {0, 0, 222}, {0, 0, 224}, {0, 0, 225}, {0, 0, 226}, {0, 0, 228}, {0, 0, 230}, {0, 0, 231}, {0, 0, 232}, {0, 0, 234}, {0, 0, 236}, {0, 0, 237}, {0, 0, 238}, {0, 0, 240}, {0, 0, 242}, {0, 0, 243}, {0, 0, 244}, {0, 0, 246}, {0, 0, 248}, {0, 0, 249}, {0, 0, 250}, {0, 0, 252}, {0, 0, 254}, {0, 0, 255}, {3, 3, 255}, {7, 7, 254}, {10, 10, 254}, {14, 14, 253}, {17, 17, 253}, {20, 20, 253}, {24, 24, 252}, {27, 27, 252}, {31, 31, 251}, {34, 34, 251}, {37, 37, 250}, {41, 41, 250}, {44, 44, 250}, {48, 48, 249}, {51, 51, 249}, {54, 54, 248}, {58, 58, 248}, {61, 61, 248}, {65, 65, 247}, {68, 68, 247}, {71, 71, 246}, {75, 75, 246}, {78, 78, 245}, {82, 82, 245}, {85, 85, 245}, {88, 88, 244}, {92, 92, 244}, {95, 95, 243}, {99, 99, 243}, {102, 102, 243}, {105, 105, 242}, {109, 109, 242}, {112, 112, 241}, {116, 116, 241}, {119, 119, 241}, {122, 122, 240}, {126, 126, 240}, {129, 129, 239}, {133, 133, 239}, {136, 136, 238}, {139, 139, 238}, {143, 143, 238}, {146, 146, 237}, {150, 150, 237}, {153, 153, 236}, {156, 156, 236}, {160, 160, 236}, {163, 163, 235}, {167, 167, 235}, {170, 170, 234}, {173, 173, 234}, {177, 177, 234}, {180, 180, 233}, {184, 184, 233}, {187, 187, 232}, {190, 190, 232}, {194, 194, 231}, {197, 197, 231}, {201, 201, 231}, {204, 204, 230}, {207, 207, 230}, {211, 211, 229}, {214, 214, 229}, {218, 218, 229}, {221, 221, 228}, {224, 224, 228}, {228, 228, 227}, {231, 231, 227}, {235, 235, 226}, {238, 238, 226}, {241, 241, 226}, {245, 245, 225}, {248, 248, 225}, {252, 252, 224}, {255, 255, 224}, {255, 255, 227}, {255, 255, 230}, {255, 255, 234}, {255, 255, 237}, {255, 255, 240}, {254, 254, 242}, {253, 253, 244}, {252, 252, 246}, {251, 251, 248}, {250, 250, 250}] ("Array 2") cluster{u8, u8, u8}[] [{0, 0, 0}, {3, 0, 0}, {6, 0, 0}, {9, 0, 0}, {12, 0, 0}, {15, 0, 0}, {18, 0, 0}, {21, 0, 0}, {24, 0, 0}, {27, 0, 0}, {30, 0, 0}, {33, 0, 0}, {36, 0, 0}, {39, 0, 0}, {42, 0, 0}, {45, 0, 0}, {48, 0, 0}, {51, 0, 0}, {54, 0, 0}, {57, 0, 0}, {60, 0, 0}, {63, 0, 0}, {66, 0, 0}, {69, 0, 0}, {72, 0, 0}, {75, 0, 0}, {78, 0, 0}, {81, 0, 0}, {84, 0, 0}, {87, 0, 0}, {90, 0, 0}, {93, 0, 0}, {96, 0, 0}, {99, 0, 0}, {102, 0, 0}, {105, 0, 0}, {108, 0, 0}, {111, 0, 0}, {114, 0, 0}, {117, 0, 0}, {120, 0, 0}, {123, 0, 0}, {126, 0, 0}, {129, 0, 0}, {132, 0, 0}, {135, 0, 0}, {138, 0, 0}, {141, 0, 0}, {144, 0, 0}, {147, 0, 0}, {150, 0, 0}, {153, 0, 0}, {156, 0, 0}, {159, 0, 0}, {162, 0, 0}, {165, 0, 0}, {168, 0, 0}, {171, 0, 0}, {174, 0, 0}, {177, 0, 0}, {180, 0, 0}, {183, 0, 0}, {186, 0, 0}, {189, 0, 0}, {192, 0, 0}, {195, 0, 0}, {198, 0, 0}, {201, 0, 0}, {204, 0, 0}, {207, 0, 0}, {210, 0, 0}, {213, 0, 0}, {216, 0, 0}, {219, 0, 0}, {222, 0, 0}, {225, 0, 0}, {228, 0, 0}, {231, 0, 0}, {234, 0, 0}, {237, 0, 0}, {240, 0, 0}, {243, 0, 0}, {246, 0, 0}, {249, 0, 0}, {252, 0, 0}, {255, 0, 0}, {255, 3, 0}, {255, 6, 0}, {255, 9, 0}, {255, 12, 0}, {255, 15, 0}, {255, 18, 0}, {255, 21, 0}, {255, 24, 0}, {255, 27, 0}, {255, 30, 0}, {255, 33, 0}, {255, 36, 0}, {255, 39, 0}, {255, 42, 0}, {255, 45, 0}, {255, 48, 0}, {255, 51, 0}, {255, 54, 0}, {255, 57, 0}, {255, 60, 0}, {255, 63, 0}, {255, 66, 0}, {255, 69, 0}, {255, 72, 0}, {255, 75, 0}, {255, 78, 0}, {255, 81, 0}, {255, 84, 0}, {255, 87, 0}, {255, 90, 0}, {255, 93, 0}, {255, 96, 0}, {255, 100, 0}, {255, 103, 0}, {255, 106, 0}, {255, 109, 0}, {255, 112, 0}, {255, 115, 0}, {255, 118, 0}, {255, 121, 0}, {255, 124, 0}, {255, 127, 0}, {255, 130, 0}, {255, 132, 0}, {255, 135, 0}, {255, 137, 0}, {255, 140, 0}, {255, 143, 0}, {255, 146, 0}, {255, 149, 0}, {255, 152, 0}, {255, 156, 0}, {255, 159, 0}, {255, 162, 0}, {255, 165, 0}, {255, 168, 0}, {255, 171, 0}, {255, 174, 0}, {255, 177, 0}, {255, 180, 0}, {255, 183, 0}, {255, 186, 0}, {255, 189, 0}, {255, 191, 0}, {255, 194, 0}, {255, 197, 0}, {255, 200, 0}, {255, 203, 0}, {255, 206, 0}, {255, 209, 0}, {255, 212, 0}, {255, 215, 0}, {255, 218, 0}, {255, 221, 0}, {255, 224, 0}, {255, 227, 0}, {255, 230, 0}, {255, 233, 0}, {255, 237, 0}, {255, 240, 0}, {255, 243, 0}, {255, 246, 0}, {255, 249, 0}, {255, 252, 0}, {255, 255, 0}, {255, 255, 3}, {255, 255, 6}, {255, 255, 9}, {255, 255, 12}, {255, 255, 15}, {255, 255, 18}, {255, 255, 21}, {255, 255, 24}, {255, 255, 27}, {255, 255, 30}, {255, 255, 33}, {255, 255, 36}, {255, 255, 39}, {255, 255, 42}, {255, 255, 45}, {255, 255, 48}, {255, 255, 51}, {255, 255, 54}, {255, 255, 57}, {255, 255, 60}, {255, 255, 63}, {255, 255, 66}, {255, 255, 69}, {255, 255, 72}, {255, 255, 75}, {255, 255, 78}, {255, 255, 81}, {255, 255, 84}, {255, 255, 87}, {255, 255, 90}, {255, 255, 93}, {255, 255, 96}, {255, 255, 99}, {255, 255, 102}, {255, 255, 105}, {255, 255, 108}, {255, 255, 111}, {255, 255, 113}, {255, 255, 116}, {255, 255, 119}, {255, 255, 122}, {255, 255, 125}, {255, 255, 128}, {255, 255, 131}, {255, 255, 134}, {255, 255, 137}, {255, 255, 140}, {255, 255, 143}, {255, 255, 146}, {255, 255, 149}, {255, 255, 152}, {255, 255, 155}, {255, 255, 158}, {255, 255, 161}, {255, 255, 164}, {255, 255, 167}, {255, 255, 170}, {255, 255, 173}, {255, 255, 176}, {255, 255, 179}, {255, 255, 182}, {255, 255, 185}, {255, 255, 188}, {255, 255, 191}, {255, 255, 194}, {255, 255, 197}, {255, 255, 200}, {255, 255, 203}, {255, 255, 206}, {255, 255, 209}, {255, 255, 212}, {255, 255, 215}, {255, 255, 218}, {255, 255, 221}, {255, 255, 224}, {255, 255, 227}, {255, 255, 230}, {255, 255, 234}, {255, 255, 237}, {255, 255, 240}, {255, 255, 243}, {255, 255, 246}, {255, 255, 249}, {255, 255, 252}, {255, 255, 255}] ("Array 2") cluster{u8, u8, u8}[] [{0, 0, 0}, {2, 0, 0}, {3, 0, 0}, {5, 0, 0}, {7, 0, 0}, {9, 0, 0}, {11, 0, 0}, {13, 0, 3}, {15, 0, 3}, {17, 0, 3}, {19, 0, 3}, {21, 0, 3}, {23, 0, 3}, {25, 0, 3}, {27, 0, 3}, {27, 0, 7}, {31, 0, 7}, {33, 0, 7}, {35, 0, 7}, {37, 0, 7}, {39, 0, 7}, {41, 0, 7}, {43, 0, 7}, {45, 0, 7}, {47, 0, 11}, {49, 0, 11}, {51, 0, 11}, {53, 0, 11}, {55, 0, 11}, {57, 0, 11}, {59, 0, 11}, {59, 3, 11}, {63, 3, 11}, {65, 3, 11}, {67, 3, 11}, {69, 3, 11}, {71, 3, 15}, {73, 3, 15}, {75, 3, 15}, {79, 3, 15}, {81, 3, 15}, {83, 3, 15}, {85, 3, 15}, {87, 3, 15}, {87, 7, 15}, {91, 7, 15}, {93, 7, 15}, {95, 7, 15}, {97, 7, 15}, {99, 7, 15}, {101, 7, 15}, {103, 7, 15}, {105, 7, 15}, {107, 11, 15}, {109, 11, 15}, {111, 11, 15}, {113, 11, 15}, {115, 11, 15}, {117, 11, 15}, {119, 11, 15}, {123, 11, 15}, {125, 11, 15}, {127, 15, 15}, {129, 15, 15}, {131, 15, 19}, {133, 15, 19}, {135, 15, 19}, {137, 15, 19}, {139, 15, 19}, {139, 19, 19}, {143, 19, 19}, {145, 19, 19}, {147, 19, 19}, {149, 19, 19}, {151, 23, 19}, {153, 23, 19}, {155, 23, 19}, {156, 23, 19}, {157, 23, 19}, {159, 27, 19}, {161, 27, 19}, {163, 27, 19}, {165, 27, 19}, {166, 31, 19}, {167, 31, 19}, {169, 31, 19}, {171, 31, 19}, {171, 35, 19}, {175, 35, 19}, {176, 35, 19}, {177, 35, 19}, {179, 39, 19}, {180, 39, 19}, {181, 39, 19}, {183, 43, 19}, {185, 43, 19}, {187, 43, 19}, {187, 47, 19}, {189, 47, 19}, {191, 47, 19}, {191, 51, 19}, {192, 51, 19}, {191, 51, 19}, {195, 55, 19}, {195, 57, 19}, {195, 59, 19}, {199, 59, 19}, {199, 61, 19}, {199, 63, 19}, {201, 63, 19}, {203, 67, 19}, {204, 67, 19}, {205, 69, 19}, {207, 71, 19}, {207, 73, 19}, {207, 75, 19}, {207, 77, 19}, {209, 79, 19}, {211, 79, 19}, {211, 83, 19}, {211, 85, 19}, {211, 87, 19}, {213, 87, 19}, {215, 91, 19}, {215, 93, 19}, {215, 95, 19}, {215, 97, 19}, {217, 99, 19}, {219, 99, 19}, {219, 103, 19}, {219, 105, 19}, {219, 106, 19}, {219, 107, 19}, {219, 111, 19}, {221, 111, 19}, {223, 115, 19}, {223, 117, 23}, {223, 119, 23}, {223, 121, 23}, {223, 123, 23}, {223, 125, 23}, {225, 127, 23}, {227, 127, 23}, {227, 131, 23}, {227, 133, 27}, {227, 135, 27}, {227, 137, 27}, {227, 139, 27}, {227, 141, 29}, {229, 143, 31}, {231, 143, 31}, {231, 145, 31}, {231, 147, 31}, {231, 149, 31}, {231, 151, 35}, {231, 153, 35}, {231, 155, 35}, {233, 157, 35}, {235, 159, 37}, {235, 160, 39}, {235, 161, 39}, {235, 163, 39}, {235, 165, 43}, {235, 167, 43}, {235, 169, 45}, {235, 171, 47}, {235, 171, 47}, {237, 173, 47}, {239, 175, 49}, {239, 177, 51}, {239, 179, 51}, {239, 179, 53}, {239, 179, 55}, {239, 183, 59}, {239, 185, 59}, {239, 187, 61}, {239, 187, 63}, {239, 189, 65}, {241, 191, 67}, {243, 191, 69}, {243, 191, 71}, {243, 191, 73}, {243, 191, 75}, {243, 197, 75}, {243, 199, 79}, {243, 201, 81}, {243, 203, 83}, {243, 203, 85}, {243, 205, 87}, {243, 207, 87}, {243, 207, 91}, {245, 209, 93}, {247, 211, 95}, {247, 211, 97}, {247, 213, 99}, {247, 215, 103}, {247, 215, 105}, {247, 215, 107}, {247, 219, 107}, {247, 219, 111}, {247, 221, 113}, {247, 223, 115}, {247, 223, 119}, {247, 223, 121}, {247, 223, 123}, {247, 227, 123}, {247, 227, 127}, {247, 227, 129}, {247, 229, 131}, {247, 231, 135}, {249, 231, 135}, {251, 231, 139}, {251, 231, 143}, {251, 235, 143}, {251, 235, 147}, {251, 235, 149}, {251, 235, 151}, {251, 237, 153}, {251, 239, 155}, {251, 239, 159}, {251, 239, 161}, {251, 239, 163}, {251, 241, 167}, {251, 243, 167}, {251, 243, 171}, {251, 243, 173}, {251, 243, 175}, {251, 243, 179}, {251, 245, 181}, {251, 247, 183}, {251, 247, 187}, {251, 247, 189}, {251, 247, 191}, {251, 247, 193}, {251, 247, 195}, {251, 247, 199}, {251, 249, 201}, {251, 251, 203}, {251, 251, 207}, {251, 251, 209}, {251, 251, 211}, {251, 251, 213}, {251, 251, 215}, {251, 251, 219}, {251, 251, 221}, {251, 251, 223}, {251, 251, 227}, {251, 251, 229}, {251, 251, 231}, {251, 251, 235}, {251, 251, 237}, {251, 251, 239}, {251, 251, 243}, {251, 251, 245}, {251, 251, 247}, {251, 251, 251}] ("Array")] -> w304
              frame "Gray", Default {
              }
              frame "Red" {
              }
              frame "Green" {
              }
              frame "Blue" {
              }
              frame "Cyan" {
              }
              frame "Magenta" {
              }
              frame "Yellow" {
              }
              frame "Red-White" {
              }
              frame "Green-White" {
              }
              frame "Blue-White" {
              }
              frame "Fire" {
              }
              frame "Glow" {
              }
            }
            n170 = To More Specific Class(target class=w309, reference=w308) -> (specific class reference=w307:refnum<vi>)  [unwired: 1 in, 1 out]
            n171 = property class="ImageControl"(reference=w307, "Palette Type"=w305) -> (reference out=w306:refnum<vi>)  [unwired: 1 in, 1 out]
            n172 = property class="ImageControl"(reference=w317, "User Palette"=w304) -> ()  [unwired: 1 in, 2 out]
            n173 = property class="ImageControl"(reference=w306, "User Palette"=w304) -> ()  [unwired: 1 in, 2 out]
          }
          frame "Line Tool", "Pan Tool", "Point Tool", "Rectangle Tool", "Zoom Tool" {
            w338 = u32 0 items=["Zoom Tool"=8, "Selection Tool"=0, "Pan Tool"=9, "Point Tool"=1, "Line Tool"=2, "Rectangle Tool"=3, "Rotated Rectangle Tool"=12, "Polyline Tool"=10, "Polygon Tool"=5, "Freehand Tool"=11, "Closed Freehand Tool"=6, "Ellipse Tool"=4, "Annulus Tool"=7] ("Current ROI Tool")
            n174 = case shown="\"Point Tool\"" w335 {
              tunnel: [w342 w343 w344 w345 w346 w347] -> w334
              frame Default {
                w342 = u32 0 items=["Zoom Tool"=8, "Selection Tool"=0, "Pan Tool"=9, "Point Tool"=1, "Line Tool"=2, "Rectangle Tool"=3, "Rotated Rectangle Tool"=12, "Polyline Tool"=10, "Polygon Tool"=5, "Freehand Tool"=11, "Closed Freehand Tool"=6, "Ellipse Tool"=4, "Annulus Tool"=7] ("Current ROI Tool")
              }
              frame "Line Tool" {
                w343 = u32 2 items=["Zoom Tool"=8, "Selection Tool"=0, "Pan Tool"=9, "Point Tool"=1, "Line Tool"=2, "Rectangle Tool"=3, "Rotated Rectangle Tool"=12, "Polyline Tool"=10, "Polygon Tool"=5, "Freehand Tool"=11, "Closed Freehand Tool"=6, "Ellipse Tool"=4, "Annulus Tool"=7] ("Current ROI Tool")
              }
              frame "Pan Tool" {
                w344 = u32 9 items=["Zoom Tool"=8, "Selection Tool"=0, "Pan Tool"=9, "Point Tool"=1, "Line Tool"=2, "Rectangle Tool"=3, "Rotated Rectangle Tool"=12, "Polyline Tool"=10, "Polygon Tool"=5, "Freehand Tool"=11, "Closed Freehand Tool"=6, "Ellipse Tool"=4, "Annulus Tool"=7] ("Current ROI Tool")
              }
              frame "Point Tool" {
                w345 = u32 1 items=["Zoom Tool"=8, "Selection Tool"=0, "Pan Tool"=9, "Point Tool"=1, "Line Tool"=2, "Rectangle Tool"=3, "Rotated Rectangle Tool"=12, "Polyline Tool"=10, "Polygon Tool"=5, "Freehand Tool"=11, "Closed Freehand Tool"=6, "Ellipse Tool"=4, "Annulus Tool"=7] ("Current ROI Tool")
              }
              frame "Rectangle Tool" {
                w346 = u32 3 items=["Zoom Tool"=8, "Selection Tool"=0, "Pan Tool"=9, "Point Tool"=1, "Line Tool"=2, "Rectangle Tool"=3, "Rotated Rectangle Tool"=12, "Polyline Tool"=10, "Polygon Tool"=5, "Freehand Tool"=11, "Closed Freehand Tool"=6, "Ellipse Tool"=4, "Annulus Tool"=7] ("Current ROI Tool")
              }
              frame "Zoom Tool" {
                w347 = u32 8 items=["Zoom Tool"=8, "Selection Tool"=0, "Pan Tool"=9, "Point Tool"=1, "Line Tool"=2, "Rectangle Tool"=3, "Rotated Rectangle Tool"=12, "Polyline Tool"=10, "Polygon Tool"=5, "Freehand Tool"=11, "Closed Freehand Tool"=6, "Ellipse Tool"=4, "Annulus Tool"=7] ("Current ROI Tool")
              }
            }
            n175 = property class="ImageControl"(reference=w341) -> (reference out=w337:refnum<vi>, "Current ROI Tool"=w340:u32)  [unwired: 1 in, 1 out]
            n176 = Equal?(x=w340, y=w334) -> (x = y?=w339:bool)
            n177 = Select(t=w338, s=w339, f=w334) -> (s? t:f=w336:u32)
            n178 = property class="ImageControl"(reference=w337, "Current ROI Tool"=w336) -> ()  [unwired: 1 in, 2 out]
          }
          frame "Auto Scale Z" {
            w372 = u32 14 items=["Default"=10, "Most Significant Bits"=11, "Full Dynamic"=12, "Downshift"=13, "Given Range"=14, "90% Dynamic"=15, "Given Percent Range"=16] ("16-bit Display Mapping:Conversion Method")
            w371 = u32 10 items=["Default"=10, "Most Significant Bits"=11, "Full Dynamic"=12, "Downshift"=13, "Given Range"=14, "90% Dynamic"=15, "Given Percent Range"=16] ("16-bit Display Mapping:Conversion Method")
            n179 = for {
              tunnel: w369 -> [w377] mode=indexing
              tunnel: w366 -> [w378]
              tunnel: [w376] -> w367
              i -> [w376]
              stop <- w379 stop-if-true
              n180 = Equal?(x=w378, y=w377) -> (x = y?=w379:bool)
            }
            n181 = property class="ImageControl"(reference=w366) -> (reference out=w375:refnum<vi>, "16-bit Display Conversion Method"=w374:u32, "Value"=w356:variant)  [unwired: 1 in, 1 out]
            n182 = Index Array(array=w368, index=w367) -> (element=w365:refnum<vi>)
            n183 = property class="Clust (strict)"(reference=w365) -> ("Controls[]"=w364:refnum<vi>[])  [unwired: 1 in, 2 out]
            n184 = Variant To Data(type=T3 refnum ("New Image"), Variant=w356) -> (data=w354:T3)  [unwired: 1 in, 1 out]
            n185 = call "IMAQ Quantify 2"("Image"=w354) -> ("Global Report"=w355:T16)  [unwired: 8 in, 2 out]
            n186 = Equal?(x=w374, y=w371) -> (x = y?=w373:bool)
            n187 = Unbundle By Name(w355) -> ("Maximal Value"=w351:sgl, "Minimal Value"=w350:sgl)
            n188 = Select(t=w372, s=w373, f=w371) -> (s? t:f=w370:u32)
            n189 = To Long Integer(number=w351) -> (32bit integer=w353:i32)
            n190 = To Long Integer(number=w350) -> (32bit integer=w352:i32)
            n191 = To Single Precision Float(number=w351) -> (single precision float=w348:sgl)
            n192 = To Single Precision Float(number=w350) -> (single precision float=w349:sgl)
            n193 = property class="ImageControl"(reference=w375, "16-bit Display Conversion Method"=w370, "16-bit Display Maximum Value"=w353, "16-bit Display Minimum Value"=w352) -> ()  [unwired: 1 in, 2 out]
            n194 = Index Array(array=w364, index #1=2 ("index"), index #2=1 ("index")) -> (element #1=w361:refnum<vi>, element #2=w358:refnum<vi>)
            n195 = To Variant(anything=w348) -> (Variant=w360:variant)
            n196 = To Variant(anything=w349) -> (Variant=w359:variant)
            n197 = property class="Ctl"(reference=w361, "Value"=w360) -> ()  [unwired: 1 in, 2 out]
            n198 = property class="Ctl"(reference=w358, "Value"=w359) -> ()  [unwired: 1 in, 2 out]
          }
          frame "Auto Scale All" {
            n199 = for {
              tunnel: w380 -> [w382] mode=indexing
              w381 = u32 10 items=["Default"=10, "Most Significant Bits"=11, "Full Dynamic"=12, "Downshift"=13, "Given Range"=14, "90% Dynamic"=15, "Given Percent Range"=16] ("16-bit Display Mapping:Conversion Method")
              n200 = property class="ImageControl"(reference=w382, "16-bit Display Conversion Method"=w381) -> ()  [unwired: 1 in, 2 out]
            }
          }
          frame "Show Z Scale" {
            n201 = for {
              tunnel: w390 -> [w394] mode=indexing
              tunnel: w388 -> [w392]
              tunnel: [w391] -> w387
              i -> [w391]
              stop <- w393 stop-if-true
              n202 = Equal?(x=w392, y=w394) -> (x = y?=w393:bool)
            }
            n203 = Index Array(array=w389, index=w387) -> (element=w386:refnum<vi>)
            n204 = property class="Clust (strict)"(reference=w386) -> (reference out=w385:refnum<vi>, "Visible"=w384:bool)  [unwired: 1 in, 1 out]
            n205 = Not(x=w384) -> (.not. x?=w383:bool)
            n206 = property class="Clust (strict)"(reference=w385, "Visible"=w383) -> ()  [unwired: 1 in, 2 out]
          }
          frame "Lock All AutoScale" {
            n207 = call "Lock Displays AE.vi"("Action"=Standard_Action."Read") -> ("Lock All Markers Out"=w400:bool, "Lock All AutoScale Out"=w398:bool, "Lock Pan/Zoom Out"=w397:bool)  [unwired: 12 in]
            n208 = Not(x=w398) -> (.not. x?=w399:bool)
            n209 = call "Lock Displays AE.vi"("Lock All Markers"=w400, "Action"=Standard_Action."Write", "Lock All AutoScale"=w399, "Lock Pan/Zoom"=w397) -> ()  [unwired: 9 in, 3 out]
          }
          frame "Lock All Markers" {
            n210 = property class="ImageControl"(reference=w402) -> ("ROI"=w403:T12)  [unwired: 1 in, 2 out]
            n211 = call "Lock Displays AE.vi"("Action"=Standard_Action."Read") -> ("Lock All Markers Out"=w407:bool, "Lock All AutoScale Out"=w404:bool, "Lock Pan/Zoom Out"=w409:bool)  [unwired: 12 in]
            n212 = Not(x=w407) -> (.not. x?=w408:bool)
            n213 = call "Lock Displays AE.vi"("Lock All Markers"=w408, "Action"=Standard_Action."Write", "Lock All AutoScale"=w404, "Lock Pan/Zoom"=w409) -> ()  [unwired: 9 in, 3 out]
            n214 = for {
              tunnel: w401 -> [w411] mode=indexing
              tunnel: w403 -> [w410]
              n215 = property class="ImageControl"(reference=w411, "ROI"=w410) -> ()  [unwired: 1 in, 2 out]
            }
          }
          frame "Lock Zoom/Pan" {
            n216 = property class="ImageControl"(reference=w412) -> ("ZoomSingle"=w415:cluster{"X":sgl, "Y":sgl}, "Image Center Position"=w414:cluster{"X":u32, "Y":u32})  [unwired: 1 in, 2 out]
            n217 = call "Lock Displays AE.vi"("Action"=Standard_Action."Read") -> ("Lock All Markers Out"=w419:bool, "Lock All AutoScale Out"=w418:bool, "Lock Pan/Zoom Out"=w416:bool)  [unwired: 12 in]
            n218 = Not(x=w416) -> (.not. x?=w417:bool)
            n219 = call "Lock Displays AE.vi"("Lock All Markers"=w419, "Action"=Standard_Action."Write", "Lock All AutoScale"=w418, "Lock Pan/Zoom"=w417) -> ()  [unwired: 9 in, 3 out]
            n220 = for {
              tunnel: w413 -> [w424] mode=indexing
              tunnel: w415 -> [w423]
              tunnel: w414 -> [w422]
              n221 = property class="ImageControl"(reference=w424, "ZoomSingle"=w423, "Image Center Position"=w422) -> ()  [unwired: 1 in, 2 out]
            }
          }
          frame "Clear All Markers", "Clear Markers" {
            n222 = Build Array(w429) -> (w428:refnum<vi>[])
            n223 = Equal?(x="Clear Markers", y=w431) -> (x = y?=w426:bool)
            n224 = Select(t=w428, s=w426, f=w427) -> (s? t:f=w425:refnum<vi>[])
            n225 = for {
              tunnel: w425 -> [w432] mode=indexing
              n226 = property class="ImageControl"(reference=w432, "ROI"=T12 {"Global Rectangle"=[], "Contours"=[]}) -> ("Value"=w433:variant)  [unwired: 1 in, 2 out]
              n227 = Variant To Data(type=T3 refnum ("New Image"), Variant=w433) -> (data=w436:T3)  [unwired: 1 in, 1 out]
              n228 = Not A Number/Path/Refnum?(number/path/refnum=w436) -> (NaN/Path/Refnum?=w435:bool)
              n229 = case shown="False" w435 {
                tunnel: w436 -> [w444 _]
                frame False {
                  w438 = "Image ROI" ("element")
                  n230 = call "IMAQ Clear Overlay"("Image"=w444) -> ("Image Out"=w443:T3)  [unwired: 9 in, 1 out]
                  n231 = call "IMAQ Get Custom Keys"("Image"=w443) -> ("Keys"=w442:string[], "Image (duplicate)"=w439:T3)  [unwired: 7 in, 2 out]
                  n232 = Search 1D Array(1D array=w442, element=w438) -> (index of element=w441:i32)  [unwired: 1 in]
                  n233 = Less Than 0?(x=w441) -> (x < 0?=w440:bool)
                  n234 = case shown="False" w440 {
                    tunnel: w439 -> [w446 _]
                    tunnel: w438 -> [w445 _]
                    frame False {
                      n235 = call "IMAQ Remove Custom Data"("Key"=w445, "Image"=w446) -> ()  [unwired: 7 in, 3 out]
                    }
                    frame True {
                    }
                  }
                }
                frame True {
                }
              }
            }
          }
          frame "Reset Zoom" {
            n236 = call "Lock Displays AE.vi"("Action"=Standard_Action."Read") -> ("Lock Pan/Zoom Out"=w451:bool)  [unwired: 12 in, 2 out]
            n237 = Build Array(w453) -> (w448:refnum<vi>[])
            n238 = Not(x=w451) -> (.not. x?=w450:bool)
            n239 = Select(t=w448, s=w450, f=w449) -> (s? t:f=w447:refnum<vi>[])
            n240 = for {
              tunnel: w447 -> [w457] mode=indexing
              w454 = u32 0 items=["Zoom Tool"=8, "Selection Tool"=0, "Pan Tool"=9, "Point Tool"=1, "Line Tool"=2, "Rectangle Tool"=3, "Rotated Rectangle Tool"=12, "Polyline Tool"=10, "Polygon Tool"=5, "Freehand Tool"=11, "Closed Freehand Tool"=6, "Ellipse Tool"=4, "Annulus Tool"=7] ("Current ROI Tool")
              n241 = property class="ImageControl"(reference=w457, "Zoom to Fit Mode"=TRUE) -> (reference out=w455:refnum<vi>)  [unwired: 1 in, 1 out]
              n242 = property class="ImageControl"(reference=w455, "Current ROI Tool"=w454) -> ()  [unwired: 1 in, 2 out]
            }
          }
          frame "Merge Tool" {
            n243 = control-ref of="This VI"() -> (w458:refnum<vi>)
            n244 = call "Display Module - Run Merge Tool.vi"("Calling VI Ref"=w458) -> ()  [unwired: 15 in]
          }
          frame "Load Image" {
          }
          frame "Save Image" {
            n245 = property class="ImageControl"(reference=w462) -> ("Value"=w461:variant)  [unwired: 1 in, 2 out]
            n246 = Variant To Data(type=T3 refnum ("Image"), Variant=w461) -> (data=w459:T3)  [unwired: 1 in, 1 out]
            n247 = call "File Dialog"("prompt"="Save TIF Image", "button label"="Save", "pattern (all files)"="*.tif", "pattern label"="TIF") -> ("selected path"=w463:path, "error out"=w464:errorcluster)  [unwired: 8 in, 2 out]
            n248 = case shown="No Error" w464 {
              tunnel: w463 -> [w487 _]
              tunnel: w459 -> [w488 _]
              frame No Error {
                w471 = 0.0 ("Z Step (µm)")
                w472 = u32 1 ("No. of Frames")
                w473 = 1.0 ("Pixel Height (µm)")
                n249 = call "IMAQ ImageToArray"("Image"=w488) -> ("Image Pixels (U16)"=w470:u16[][])  [unwired: 3 in, 4 out]
                n250 = Array Size(array=w470) -> (size(s)=w479:i32[])
                n251 = To Unsigned Long Integer(number=w479) -> (unsigned 32bit integer=w469:u32[])
                n252 = Index Array(array=w469, index #1=1 ("index"), index #2=0 ("index")) -> (element #1=w476:u32, element #2=w475:u32)
                n253 = Bundle By Name(cluster=T13 {"Image Width (Pixels)"=0, "Image Height (Pixels)"=0, "Pixel Width (µm)"=0.0, "Pixel Height (µm)"=0.0, "Bits Per Sample (e.g. 16)"=0, "No. of Frames"=0, "No. of Slices"=0, "Time Step (sec)"=0.0, "Z Step (µm)"=0.0} ("Image Info"), "Image Width (Pixels)"=w476, "Image Height (Pixels)"=w475, "Pixel Width (µm)"=w473, "Pixel Height (µm)"=w473, "Bits Per Sample (e.g. 16)"=u32 16, "No. of Frames"=w472, "No. of Slices"=w472, "Time Step (sec)"=w471, "Z Step (µm)"=w471) -> (w480:T13)
                n254 = call "Write TIFF Header.vi"("File Path"=w487, "Image Info"=w480) -> ("File Ref"=w486:refnum<file>, "Byte Order"=w482:T17, "Error"=w483:errorcluster)  [unwired: 11 in]
                n255 = Write to Binary File(file (use dialog)=w486, data=w470, error in=w483, 9:w482) -> (refnum out=w485:refnum<file>, error out=w484:errorcluster)  [unwired: 2 in, 1 out]
                n256 = Close File(refnum=w485, error in=w484) -> ()  [unwired: 2 out]
              }
              frame Error {
              }
            }
          }
        }
      }
      event "Channel 1", "Channel 2", "Channel 3", "Channel 4", "Channel 5", "Channel 6": Mouse Up {
        # "1: Left Click\n2: Right Click\n3: Middle Click"
        n257 = event-data() -> ("CtlRef"=w490:refnum<vi>)  [unwired: 1 in, 1 out]
        n258 = property class="ImageControl"(reference=w490) -> ("ZoomSingle"=w498:cluster{"X":sgl, "Y":sgl}, "Image Center Position"=w494:cluster{"X":u32, "Y":u32})  [unwired: 1 in, 2 out]
        n259 = property class="ImageControl"(reference=w490) -> ("ROI"=w491:T12)  [unwired: 1 in, 2 out]
        n260 = call "Lock Displays AE.vi"("Action"=Standard_Action."Read") -> ("Lock Pan/Zoom Out"=w495:bool)  [unwired: 12 in, 2 out]
        n261 = call "Lock Displays AE.vi"("Action"=Standard_Action."Read") -> ("Lock All Markers Out"=w499:bool)  [unwired: 12 in, 2 out]
        n262 = case shown="True" w495 {
          tunnel: w496 -> [_ w511]
          tunnel: w498 -> [_ w510]
          tunnel: w494 -> [_ w509]
          frame False {
          }
          frame True {
            n263 = for {
              tunnel: w511 -> [w514] mode=indexing
              tunnel: w510 -> [w513]
              tunnel: w509 -> [w512]
              n264 = property class="ImageControl"(reference=w514, "ZoomSingle"=w513, "Image Center Position"=w512) -> ()  [unwired: 1 in, 2 out]
            }
          }
        }
        n265 = case shown="True" w499 {
          tunnel: w496 -> [_ w516]
          tunnel: w491 -> [_ w515]
          frame False {
          }
          frame True {
            n266 = for {
              tunnel: w516 -> [w518] mode=indexing
              tunnel: w515 -> [w517]
              n267 = property class="ImageControl"(reference=w518, "ROI"=w517) -> ()  [unwired: 1 in, 2 out]
            }
          }
        }
        n268 = Unbundle By Name(w491) -> ("Contours"=w493:T18)
        n269 = Array Size(array=w493) -> (size(s)=w489:i32)
        n270 = Equal To 0?(x=w489) -> (x = 0?=w492:bool)
        n271 = case shown="False" w492 {
          tunnel: w491 -> [w508 _]
          tunnel: w490 -> [w507 _]
          frame False {
            n272 = property class="ImageControl"(reference=w507) -> ("Value"=w504:variant)  [unwired: 1 in, 2 out]
            n273 = Flatten To JSON(anything=w508) -> (JSON string=w505:string)  [unwired: 2 in, 1 out]
            n274 = Variant To Data(type=T3 refnum ("New Image"), Variant=w504) -> (data=w502:T3)  [unwired: 1 in, 1 out]
            n275 = call "IMAQ Write Custom Data"("Custom Data In"=w505, "Key"="Image ROI", "Image"=w502) -> ()  [unwired: 7 in, 2 out]
          }
          frame True {
          }
        }
      }
      event "Channel 1", "Channel 2", "Channel 3", "Channel 4", "Channel 6", "Channel 5": Mouse Enter; "Channel 1", "Channel 2", "Channel 3", "Channel 4", "Channel 5", "Channel 6": Mouse Leave {
        w519 = Standard_Action."Write" ("Action")
        n276 = event-data() -> ("Type"=w522:T11, "CtlRef"=w521:refnum<vi>)  [unwired: 1 in]
        n277 = call "Current Display Mouse.vi"("Event Type"=w522, "Action"=w519, "IMAQ Image Display Ref"=w521) -> ()  [unwired: 11 in, 2 out]
        n278 = call "Main Info Bar Message AE.vi"("Action"=w519, "Message"="") -> ()  [unwired: 13 in, 1 out]
      }
      event Value Change {
        w529 = u32 14 items=["Default"=10, "Most Significant Bits"=11, "Full Dynamic"=12, "Downshift"=13, "Given Range"=14, "90% Dynamic"=15, "Given Percent Range"=16] ("16-bit Display Mapping:Conversion Method")
        n279 = event-data() -> ("NewVal.Z Scale Max"=w526:sgl, "NewVal.Z Scale Min"=w527:sgl, "CtlRef"=w528:refnum<vi>)  [unwired: 1 in]
        n280 = for {
          tunnel: w533 -> [w535] mode=indexing
          tunnel: [w537] -> w531
          tunnel: w528 -> [w536]
          i -> [w537]
          stop <- w538 stop-if-true
          n281 = Equal?(x=w536, y=w535) -> (x = y?=w538:bool)
        }
        n282 = To Long Integer(number=w526) -> (32bit integer=w525:i32)
        n283 = To Long Integer(number=w527) -> (32bit integer=w524:i32)
        n284 = Index Array(array=w532, index=w531) -> (element=w530:refnum<vi>)
        n285 = property class="ImageControl"(reference=w530, "16-bit Display Maximum Value"=w525, "16-bit Display Minimum Value"=w524, "16-bit Display Conversion Method"=w529) -> ()  [unwired: 1 in, 2 out]
      }
      event Key Down; Key Up {
        # "Switch to the Pan Tool when the space bar is held down"
        n286 = event-data() -> ("Type"=w545:T11, "ScanCode"=w543:i16)  [unwired: 1 in]
        n287 = Equal?(x=lveventtype."Key Down", y=w545) -> (x = y?=w539:bool)
        n288 = Equal?(x=w543, y=i16 57) -> (x = y?=w541:bool)
        n289 = case shown="True" w541 {
          tunnel: w540 -> [_ w551]
          tunnel: w539 -> [_ w550]
          frame False {
          }
          frame True {
            w548 = u32 0 items=["Zoom Tool"=8, "Selection Tool"=0, "Pan Tool"=9, "Point Tool"=1, "Line Tool"=2, "Rectangle Tool"=3, "Rotated Rectangle Tool"=12, "Polyline Tool"=10, "Polygon Tool"=5, "Freehand Tool"=11, "Closed Freehand Tool"=6, "Ellipse Tool"=4, "Annulus Tool"=7] ("Current ROI Tool")
            w549 = u32 9 items=["Zoom Tool"=8, "Selection Tool"=0, "Pan Tool"=9, "Point Tool"=1, "Line Tool"=2, "Rectangle Tool"=3, "Rotated Rectangle Tool"=12, "Polyline Tool"=10, "Polygon Tool"=5, "Freehand Tool"=11, "Closed Freehand Tool"=6, "Ellipse Tool"=4, "Annulus Tool"=7] ("Current ROI Tool")
            n290 = Select(t=w549, s=w550, f=w548) -> (s? t:f=w547:u32)
            n291 = for {
              tunnel: w551 -> [w553] mode=indexing
              tunnel: w547 -> [w552]
              n292 = property class="ImageControl"(reference=w553, "Current ROI Tool"=w552) -> ()  [unwired: 1 in, 2 out]
            }
          }
        }
      }
      event "Settings": Value Change {
        n293 = event-data() -> ("NewVal"=w554:bool, "CtlRef"=w555:refnum<vi>)  [unwired: 1 in]
        n294 = case shown="False" w554 {
          tunnel: w555 -> [_ w566]
          frame False {
            n295 = property on="Settings Menu" class="Clust (strict)"("Visible"=FALSE, "Left"=-100 ("Position:Left"), "Top"=0 ("Position:Top")) -> ()  [unwired: 2 in, 2 out]
          }
          frame True {
            n296 = property class="Bool (strict)"(reference=w566) -> ("Left"=w565:i32, "Top"=w560:i32)  [unwired: 1 in, 2 out]
            n297 = property on="Settings Menu" class="Clust (strict)"() -> ("Height"=w563:u32)  [unwired: 2 in, 2 out]
            n298 = To Long Integer(number=w563) -> (32bit integer=w561:i32)
            n299 = Subtract(x=w560, y=w561) -> (x-y=w562:i32)
            n300 = property on="Settings Menu" class="Clust (strict)"("Visible"=TRUE, "Left"=w565, "Top"=w562) -> ()  [unwired: 2 in, 2 out]
          }
        }
      }
      event "Settings Menu": Value Change {
        # "0: Refresh Rate\n1: Display Order\n2: Display On / Off"
        n301 = event-data() -> ("NewVal"=w573:T1)  [unwired: 1 in]
        n302 = local write "Settings"(FALSE ("Settings")) -> ()
        n303 = Cluster To Array(cluster=w573) -> (array=w572:bool[])
        n304 = property on="Settings Menu" class="Clust (strict)"("Visible"=FALSE, "Left"=-100 ("Position:Left"), "Top"=0 ("Position:Top"), "Value"=T1 {"Refresh Rate"=FALSE, "Change Display Order"=FALSE, "Display On / Off"=FALSE} ("Settings Menu")) -> ()  [unwired: 2 in, 2 out]
        n305 = Search 1D Array(1D array=w572, element=TRUE, start index (0)=0) -> (index of element=w569:i32)
        n306 = case shown="1" w569 {
          tunnel: w568 -> [_ _ w589 w599]
          tunnel: w567 -> [_ _ w582 w592]
          frame Default {
          }
          frame 0 {
            n307 = local read "Refresh Rate (ms)"() -> (w581:u32)
            n308 = call "Display Module Refresh Rate.vi"("Refresh Rate In"=w581) -> ("Refresh Rate Out"=w580:u32)  [unwired: 14 in]
            n309 = local write "Refresh Rate (ms)"(w580) -> ()
          }
          frame 1 {
            n310 = vi-ref "Display Module - Set Display Order.vi"() -> (w588:refnum<vi>)
            n311 = Get Notifier Status(notifier=w589) -> (current notification=w583:T3[])  [unwired: 1 in, 4 out]
            n312 = property class="VI Interface Type 0"(reference=w588) -> ("Path"=w587:path)  [unwired: 1 in, 2 out]
            n313 = Open VI Reference(type specifier VI Refnum (for type only)=w588, vi path=w587, options=128) -> (vi reference=w586:refnum<vi>)  [unwired: 3 in, 1 out]
            n314 = call-by-ref "Start Asynchronous Call"(reference=w586, "Image Refs"=w583, "IMAQ Display Refs"=w582) -> (reference out=w585:refnum<vi>)  [unwired: 15 in, 1 out]
            n315 = Close Reference(reference=w585) -> ()  [unwired: 1 in, 1 out]
          }
          frame 2 {
            n316 = Get Notifier Status(notifier=w599) -> (notifier out=w597:refnum<notifier>, current notification=w598:T3[])  [unwired: 1 in, 3 out]
            n317 = call "Display Module - All Images Active.vi"("Image Refs In"=w598) -> ("Image Refs Out"=w593:T3[])  [unwired: 14 in]
            n318 = vi-ref "Display Module - Switch On and Off.vi"() -> (w596:refnum<vi>)
            n319 = Send Notification(notification=w593, notifier=w597) -> ()  [unwired: 1 in, 2 out]
            n320 = property class="VI Interface Type 1"(reference=w596) -> ("Path"=w595:path)  [unwired: 1 in, 2 out]
            n321 = Open VI Reference(type specifier VI Refnum (for type only)=w596, vi path=w595, options=128) -> (vi reference=w594:refnum<vi>)  [unwired: 3 in, 1 out]
            n322 = call-by-ref "Start Asynchronous Call"(reference=w594, "Image Refs"=w593, "IMAQ Display Refs"=w592) -> (reference out=w591:refnum<vi>)  [unwired: 15 in, 1 out]
            n323 = Close Reference(reference=w591) -> ()  [unwired: 1 in, 1 out]
          }
        }
      }
      event "Exit": Value Change {
        n324 = event-data() -> ("NewVal"=w604:bool)  [unwired: 1 in]
        n325 = Close Reference(reference=w603) -> ()  [unwired: 1 in, 1 out]
        n326 = call "IMAQ Dispose"("Image"=w602) -> ()  [unwired: 5 in, 1 out]
        n327 = call "Main Info Bar Message AE.vi"("Action"=Standard_Action."Write", "Message"="") -> ()  [unwired: 13 in, 1 out]
      }
    }
  }
  n328 = Release Notifier(notifier=w55) -> ()  [unwired: 2 in, 3 out]
